vi "ME_acquire_14_DeltaForce_Daq_steppingMode.vi"() -> ()   [LabVIEW 2015]
doc: "Use this template to build a producer/consumer design pattern. Use this template when you need to execute a process, such as data analysis, when a data source, such as a triggered acquisition, produces data at an uneven rate and you need to execute the process when the data becomes available."
uses:
  Mode.ctl
  oxford_driver/Oxford Drivers/BUSGEN.LLB/OxfordAddress.ctl
  <vilib>/Analysis/baseanly.llb/Mean (DBL).vi
  <vilib>/DAQmx/read.llb/DAQmx Read (Analog 1D DBL 1Chan NSamp).vi
  <vilib>/DAQmx/create/channels.llb/DAQmx Create Channel (AI-Voltage-Basic).vi
  <vilib>/DAQmx/configure/timing.llb/DAQmx Timing (Sample Clock).vi
  <vilib>/Utility/file.llb/Write Delimited Spreadsheet (DBL).vi
  <vilib>/DAQmx/miscellaneous.llb/DAQmx Fill In Error Info.vi
  <vilib>/express/express arith-compare/Formula/XNode/ExpressFormulaBlockNode.xnode
  <vilib>/Analysis/NI_AALBase.lvlib
panel:
  out "No pol":bool=TRUE
  out "Actual2":dbl
  in  "First offset?":bool
  in  "Ready2Step":bool
  out "Last2":dbl
  out "remaining elements 2":T1(array[cluster])
  out "Actual mean":dbl format="%0.6f"
  in  "Averaged dt":dbl[][](array[numeric])
  in  "Averaged P(B)":dbl[][](array[numeric])
  out "LockInR":dbl
  out "deltaUaux":dbl
  out "Actual Voltage (V)":dbl caption="Actual AuxV" step=0.1
  in  "Stop":bool
  out "SaveSweep":bool=TRUE
  out "Measurement File_dn":path
  out "Measurement File_up":path
  out "Measurement File_average":path
  out "Actual Polarization":dbl
  in  "Reset IB?":bool
  in  "First?":bool
  in  "Save Period":dbl=1.0
  out "Averaged I(B)":dbl[][](array[numeric])
  out "P(uC/mm^2)":dbl[](array[numeric])
  in  "Sweep":bool
  out "Offset array":dbl[](array[numeric])
  in  "stop 2":bool
  in  "dB":dbl=0.005
  in  "Dwell Time (ms)":u32=1
  out "appended array":dbl[][](array[numeric])
  out "Actual B Field (T)":dbl
  out "Actual Temperature (K)":dbl
  out "Actual Current (pA)":dbl
  in  "Tab Control":T2(tab)
  in  "Max temperature (K)":dbl=20.0
  in  "Min Temperature (K)":dbl=4.5
  out "P(T)":cluster{"yi":dbl[], dbl[]}(graph)
  out "I(T)":cluster{dbl[], dbl[]}(graph)
  in  "Set temperature (K)":dbl=4.5
  in  "Temp Ramping Rate (K/min)":dbl=10.0
  in  "Heater Range":enum16{"Off", "Low", "Medium", "High"}(ring)
  in  "Heater On/Off":bool
  out "Setpoint Temperature (K)":dbl
  in  "Window (s)":dbl
  in  "Dwell Time (s)":dbl
  in  "Field Step (T)":dbl
  in  "Stepping Mode":bool
  out "I(B) 3":cluster{dbl[], dbl[]}[](graph)
  out "I(B) /Averaged/":cluster{"B array":dbl[], dbl[]}[](graph)
  out "P(B) /Averaged/":cluster{"B array":dbl[], dbl[]}[](graph)
  out "P(B)":cluster{"yi":dbl[], dbl[]}(graph)
  in  "Set Field (T)":dbl
  in  "Go to Set":bool
  in  "Sweep Rate (T/min)":dbl=2.0 format="%.6f"
  in  "Field To Zero":bool
  out "Target Field":dbl
  in  "Min Field (T)":dbl
  in  "Max Field (T)":dbl=0.15
  in  "Threshold B (T)":dbl
  out "Up/Down":bool
  in  "ReOffset":bool
  out "I(t)":dbl(graph)
  out "B(t)":dbl(graph)
  in  "Max count array":i32[](array[numeric])=[2, 1, 0, 0, 0, 9, 10, 11, 12]
  in  "secs to wait":dbl=180.0
  out "Wait (s)":dbl
  in  "Directory":string
  out "Finished":bool=TRUE
  out "Step Rate":bool
  out "New":bool=TRUE
  in  "Temperature Array":dbl[](array[numeric])=[4.5, 5.0, 6.0, 7.0, 8.0, 9.0, 10.0, 11.0, 12.0]
  in  "Sweep Rate Array":dbl[](array[numeric])=[2.0, 1.0, 0.5, 0.1, 0.05, 9.0, 10.0, 11.0, 12.0]
  in  "Record ALL":bool
  in  "Max Countl":i32
  out "i":i32
  out "j":i32
  out "Step Temp":bool
  in  "FileName":string
  in  "Measure Noise":bool
  in  "Cycles":i32
  in  "maximum value":dbl=10.0 format="%0.2f"
  in  "minimum value":dbl=-10.0 format="%0.2f"
  in  "physical channels":tag="Dev1/ai1"
  out "PSD (pA/Hz^1/2) Peaks Removed":cluster{"f0":dbl, "df":dbl, "magnitude":dbl[]}(graph)
  out "PSD (pA/Hz^1/2)":cluster{"f0":dbl, "df":dbl, "magnitude":dbl[]}(graph)
  out "Current (pA) Filtered":waveform(dbl)(graph)
  out "Current (pA)":dbl[](graph)
  in  "Samples per channel":i32=1000
  in  "Rate":dbl=1000.0 format="%0.2f"
  in  "Cut-Off Frequency":dbl=100.0 caption="Lower Cut-Off"
  in  "Filter On":bool
  in  "Lock_in_Amplifier":refnum<visa-resource-name>="GPIB0::5::INSTR"
  out "Dc offset":dbl
  in  "Calibrate":bool
  in  "IV converter":refnum<visa-resource-name>="GPIB0::20::INSTR"
  in  "Magnetic Field":refnum<visa-resource-name>="GPIB0::21::INSTR"
  out "Time Lag":dbl=0.0500025749206543
  in  "Lake Shore":refnum<visa-resource-name>="GPIB0::11::INSTR"
  in  "Temp Refresh (s)":dbl=0.1
  in  "Sampling rate (Hz)":dbl=10.0
  in  "Gain (V/A)":dbl=1000000000.0
  in  "Sample area (mm^2)":dbl=1.0
  out "B_V":cluster{dbl[], "Best Linear Fit":dbl[]}[](graph)=[{[-0.00824276058, -0.00825443003, -0.00321183179, 0.00231176104, 0.00884956705, 0.0149905744, 0.0216812607, 0.0279766336, 0.0349330416, 0.0411953716, 0.0480051807, 0.0542754057, 0.0609032504, 0.0669260394, 0.0738628706, 0.0800669926, 0.0863286519, 0.0933777995, 0.099599688, 0.107340216, 0.113761556, 0.118682905, 0.126619495, 0.134198466, 0.140806839, 0.147543465, 0.154230554, 0.161238153, 0.167889746, 0.174562307, 0.180709351, 0.186845666, 0.193431356, 0.20078938, 0.206999692, 0.213664344, 0.21973451, 0.22642957, 0.232505683, 0.23932268, 0.246070279, 0.252111494, 0.259500232, 0.265590936, 0.271561847, 0.279541147, 0.28623026, 0.292989935, 0.298956555, 0.305738485, 0.312378369, 0.319038606, 0.325861428, 0.331749698, 0.337772536, 0.344588307, 0.351860931, 0.358493458, 0.364558106, 0.37132097, 0.377974157], "Best Linear Fit"=[0.0, 0.0015, 0.0036, 0.0057, 0.0077, 0.0097, 0.0117, 0.0139, 0.0159, 0.0179, 0.0199, 0.0219, 0.0239, 0.0259, 0.0279, 0.0299, 0.032, 0.034, 0.036, 0.0381, 0.0401, 0.0423, 0.0443, 0.0463, 0.0484, 0.0505, 0.0525, 0.0545, 0.0567, 0.0587, 0.0607, 0.0627, 0.0647, 0.0668, 0.0687, 0.0707, 0.0727, 0.0747, 0.0767, 0.0788, 0.0808, 0.0828, 0.0849, 0.0869, 0.0889, 0.0911, 0.0932, 0.0952, 0.0972, 0.0993, 0.1015, 0.1035, 0.1055, 0.1075, 0.1095, 0.1115, 0.1136, 0.1156, 0.1176, 0.1197, 0.1217]}, {[-0.00824276058, -0.00825443003, -0.00321183179, 0.00231176104, 0.00884956705, 0.0149905744, 0.0216812607, 0.0279766336, 0.0349330416, 0.0411953716, 0.0480051807, 0.0542754057, 0.0609032504, 0.0669260394, 0.0738628706, 0.0800669926, 0.0863286519, 0.0933777995, 0.099599688, 0.107340216, 0.113761556, 0.118682905, 0.126619495, 0.134198466, 0.140806839, 0.147543465, 0.154230554, 0.161238153, 0.167889746, 0.174562307, 0.180709351, 0.186845666, 0.193431356, 0.20078938, 0.206999692, 0.213664344, 0.21973451, 0.22642957, 0.232505683, 0.23932268, 0.246070279, 0.252111494, 0.259500232, 0.265590936, 0.271561847, 0.279541147, 0.28623026, 0.292989935, 0.298956555, 0.305738485, 0.312378369, 0.319038606, 0.325861428, 0.331749698, 0.337772536, 0.344588307, 0.351860931, 0.358493458, 0.364558106, 0.37132097, 0.377974157], "Best Linear Fit"=[0.0023130671909174904, 0.0023094596731686335, 0.003868338853520157, 0.005575913689667713, 0.007597024472065889, 0.009495468101455781, 0.01156384061080984, 0.013510005123483607, 0.015660523385123023, 0.017596472947801402, 0.01970167132429517, 0.021640061563494486, 0.023689007091511245, 0.025550904457292693, 0.027695370706757948, 0.02961332572872314, 0.03154906794982551, 0.033728255921950154, 0.035651703316228106, 0.038044626045707346, 0.04002973228648501, 0.041551128227666274, 0.04400466196665122, 0.04634764063321815, 0.04839056663989068, 0.050473141042489685, 0.05254040147513078, 0.054706745027686375, 0.056763032153958, 0.05882580137083012, 0.060726111182603806, 0.06262310420927387, 0.0646590179467223, 0.06693369260375522, 0.0688535612150383, 0.07091388542740072, 0.07279042901630216, 0.07486015362026034, 0.07673853567696039, 0.07884595613562831, 0.08093192275399225, 0.08279951637127143, 0.08508368601736883, 0.08696657876578731, 0.0888124384600611, 0.09127917565619728, 0.09334706179235687, 0.09543676161017195, 0.09728129477588952, 0.09937787455012936, 0.10143054193208385, 0.1034895012822753, 0.10559872249341117, 0.10741903437915212, 0.10928094689289425, 0.11138798834340323, 0.11363626226897475, 0.11568665529283369, 0.11756149303587794, 0.11965217870770509, 0.12170895860641172]}]
  out "V_I":cluster{dbl[], "Best Linear Fit":dbl[]}[](graph)=[{[0.0, 0.013, 0.027, 0.041, 0.054, 0.069, 0.083, 0.098, 0.112, 0.125, 0.139, 0.153, 0.167, 0.181, 0.195, 0.208, 0.222, 0.237, 0.251, 0.265, 0.28, 0.294, 0.308, 0.322, 0.337, 0.351, 0.365, 0.379, 0.393, 0.408, 0.422, 0.435, 0.449, 0.463, 0.477, 0.491, 0.505, 0.518, 0.532, 0.547, 0.561, 0.575, 0.589, 0.603, 0.618, 0.632, 0.647, 0.66, 0.674, 0.689, 0.703, 0.718, 0.731, 0.745, 0.759, 0.773, 0.787, 0.802, 0.815, 0.829, 0.844], "Best Linear Fit"=[-0.00824276058, -0.00825443003, -0.00321183179, 0.00231176104, 0.00884956705, 0.0149905744, 0.0216812607, 0.0279766336, 0.0349330416, 0.0411953716, 0.0480051807, 0.0542754057, 0.0609032504, 0.0669260394, 0.0738628706, 0.0800669926, 0.0863286519, 0.0933777995, 0.099599688, 0.107340216, 0.113761556, 0.118682905, 0.126619495, 0.134198466, 0.140806839, 0.147543465, 0.154230554, 0.161238153, 0.167889746, 0.174562307, 0.180709351, 0.186845666, 0.193431356, 0.20078938, 0.206999692, 0.213664344, 0.21973451, 0.22642957, 0.232505683, 0.23932268, 0.246070279, 0.252111494, 0.259500232, 0.265590936, 0.271561847, 0.279541147, 0.28623026, 0.292989935, 0.298956555, 0.305738485, 0.312378369, 0.319038606, 0.325861428, 0.331749698, 0.337772536, 0.344588307, 0.351860931, 0.358493458, 0.364558106, 0.37132097, 0.377974157]}, {[0.0, 0.013, 0.027, 0.041, 0.054, 0.069, 0.083, 0.098, 0.112, 0.125, 0.139, 0.153, 0.167, 0.181, 0.195, 0.208, 0.222, 0.237, 0.251, 0.265, 0.28, 0.294, 0.308, 0.322, 0.337, 0.351, 0.365, 0.379, 0.393, 0.408, 0.422, 0.435, 0.449, 0.463, 0.477, 0.491, 0.505, 0.518, 0.532, 0.547, 0.561, 0.575, 0.589, 0.603, 0.618, 0.632, 0.647, 0.66, 0.674, 0.689, 0.703, 0.718, 0.731, 0.745, 0.759, 0.773, 0.787, 0.802, 0.815, 0.829, 0.844], "Best Linear Fit"=[-0.016453575077272017, -0.010376221021590415, -0.0038313781923948447, 0.002713464636800727, 0.008790818692482327, 0.01580315029519187, 0.02234799312438744, 0.02936032472709698, 0.03590516755629255, 0.04198252161197415, 0.04852736444116973, 0.05507220727036529, 0.061617050099560866, 0.06816189292875643, 0.074706735757952, 0.0807840898136336, 0.08732893264282918, 0.09434126424553871, 0.10088610707473429, 0.10743094990392986, 0.1144432815066394, 0.12098812433583496, 0.12753296716503054, 0.1340778099942261, 0.14109014159693567, 0.1476349844261312, 0.15417982725532678, 0.16072467008452238, 0.16726951291371794, 0.17428184451642745, 0.18082668734562304, 0.18690404140130465, 0.19344888423050022, 0.19999372705969579, 0.20653856988889135, 0.21308341271808692, 0.2196282555472825, 0.2257056096029641, 0.2322504524321597, 0.23926278403486922, 0.2458076268640648, 0.2523524696932603, 0.2588973125224559, 0.2654421553516515, 0.27245448695436103, 0.2789993297835566, 0.28601166138626616, 0.29208901544194776, 0.29863385827114336, 0.30564618987385284, 0.31219103270304843, 0.31920336430575796, 0.32528071836143957, 0.3318255611906351, 0.3383704040198307, 0.3449152468490263, 0.35146008967822184, 0.35847242128093143, 0.364549775336613, 0.3710946181658085, 0.3781069497685181]}]
  out "B0 (T)":dbl=0.004861251132056582
  out "B/V (T/V)":dbl=0.30914205458325855
  out "I0 (A)":dbl=-0.016453575077272017
  out "V/I (Ohm)":dbl=0.46748877351396934
  in  "Offset?":bool
  in  "Magnet":bool
  in  "Ramp":bool=TRUE
  in  "DaQ":bool
  in  "Moving average":i8=10
  in  "Sample Rate":dbl=1000.0
  in  "Number of Samples":i32=100
  in  "Physical Channel":tag="kartya/ai0"
  in  "Min Voltage":dbl=-5.0
  in  "Max Voltage":dbl=5.0
  in  "Terminal Configuration":i32(ring)=-1 items=["default"=-1, "RSE"=10083, "NRSE"=10078, "Differential"=10106, "Pseudodifferential"=12529]
  in  "Count":i32=100
  in  "Temp/Magnetic Field":bool
  out "index":i8
  out "Read?":bool
  out "Magnetic Field (T)":dbl[](array[numeric])
  out "Reset":bool
  out "Measured Current (pA)":dbl[](array[numeric])
  out "Elapsed Time (s)":dbl[](array[numeric])
  out "Start time":timestamp
  in  "Enum":T3=enum."Process"
  out "B array":dbl[](array[numeric])
  in  "dB (T)":dbl=0.0025
  in  "Counter":i8
  out "L magnet (H)":dbl
  out "R magnet (mOhm)":dbl
  out "Actual Current (R0)":dbl
  out "Actual Field (T)":dbl
  out "Temperature array":dbl[](array[numeric])
  in  "New Measurement File":bool
  out "Measurement File":path
  out "refnum out":refnum<file>
  in  "Measuring":bool
  in  "Measure /Pause":bool
  in  "stop":bool
  # "DeltaForce"
  # "Discrete"
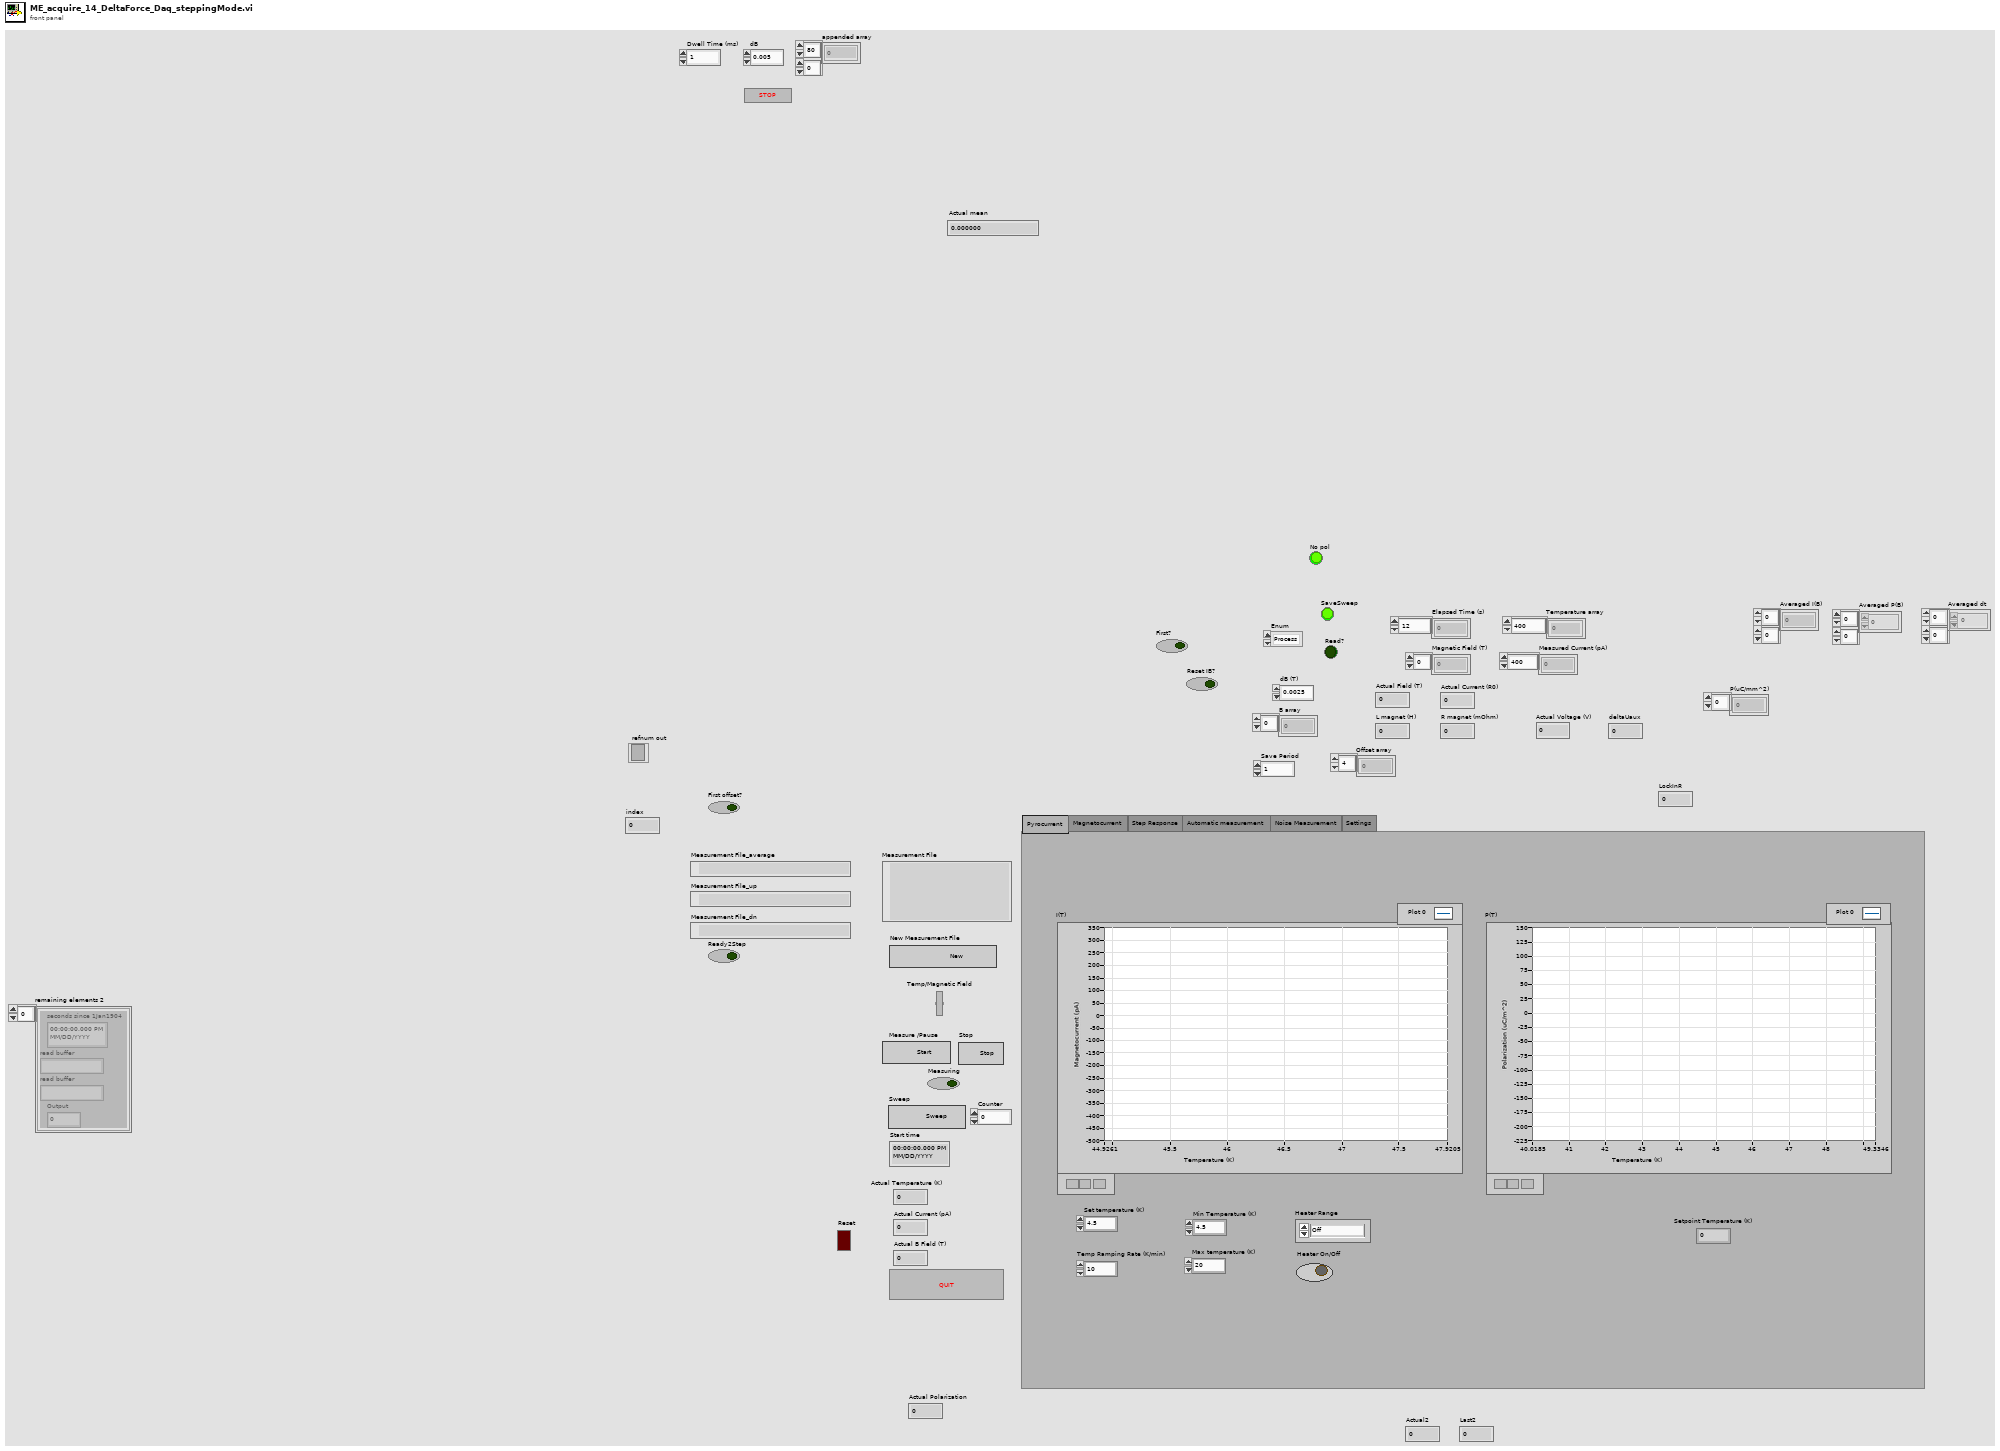
[diagram p1: front panel]
types:
  T1 = cluster{"seconds since 1Jan1904":timestamp, "read buffer":string, "read buffer":string, "Output":dbl}[]
  T2 = enum32{"Pyrocurrent", "Magnetocurrent", "Step Response", "Automatic measurement", "Noise Measurement", "Settings"}
  T3 = typedef "Mode.ctl" = enum16{"Offset", "Process", "Sweep", "StepOxford", "StepDelta", "Plot", "Save", "New", "Return", ""}
  T4 = cluster{"seconds since 1Jan1904":timestamp, "read buffer":string, "read buffer":string, "Output":dbl}
  T5 = enum16{"open", "replace", "create", "open or create", "replace or create", "replace or create with confirmation"}
  T6 = typedef "OxfordAddress.ctl" = cluster{"Com Port":i32, "ISOBUS Address":i32, "GPIB Address":i16, "Communication":enum16{"RS232", "ISOBUS", "GPIB", "Gateway"}}
  T7 = cluster{"B array":dbl[], "Averaged P(B) Out":dbl[]}
  T8 = cluster{"B array":dbl[], "BaselineSubtracted I(B)":dbl[]}
  T9 = cluster{"B array":dbl[], "Averaged P(B) Out":dbl[]}[]
  T10 = cluster{"B array":dbl[], "BaselineSubtracted I(B)":dbl[]}[]
  T11 = cluster{"I array out (A)":dbl[], "V array out (V)":dbl[]}
  T12 = cluster{"I array out (A)":dbl[], "Best Linear Fit":dbl[]}
  T13 = cluster{"V array out (V)":dbl[], "B array Out":dbl[]}
  T14 = cluster{"V array out (V)":dbl[], "Best Linear Fit 2":dbl[]}
  T15 = cluster{"I array out (A)":dbl[], "Best Linear Fit":dbl[]}[]
  T16 = cluster{"V array out (V)":dbl[], "Best Linear Fit 2":dbl[]}[]
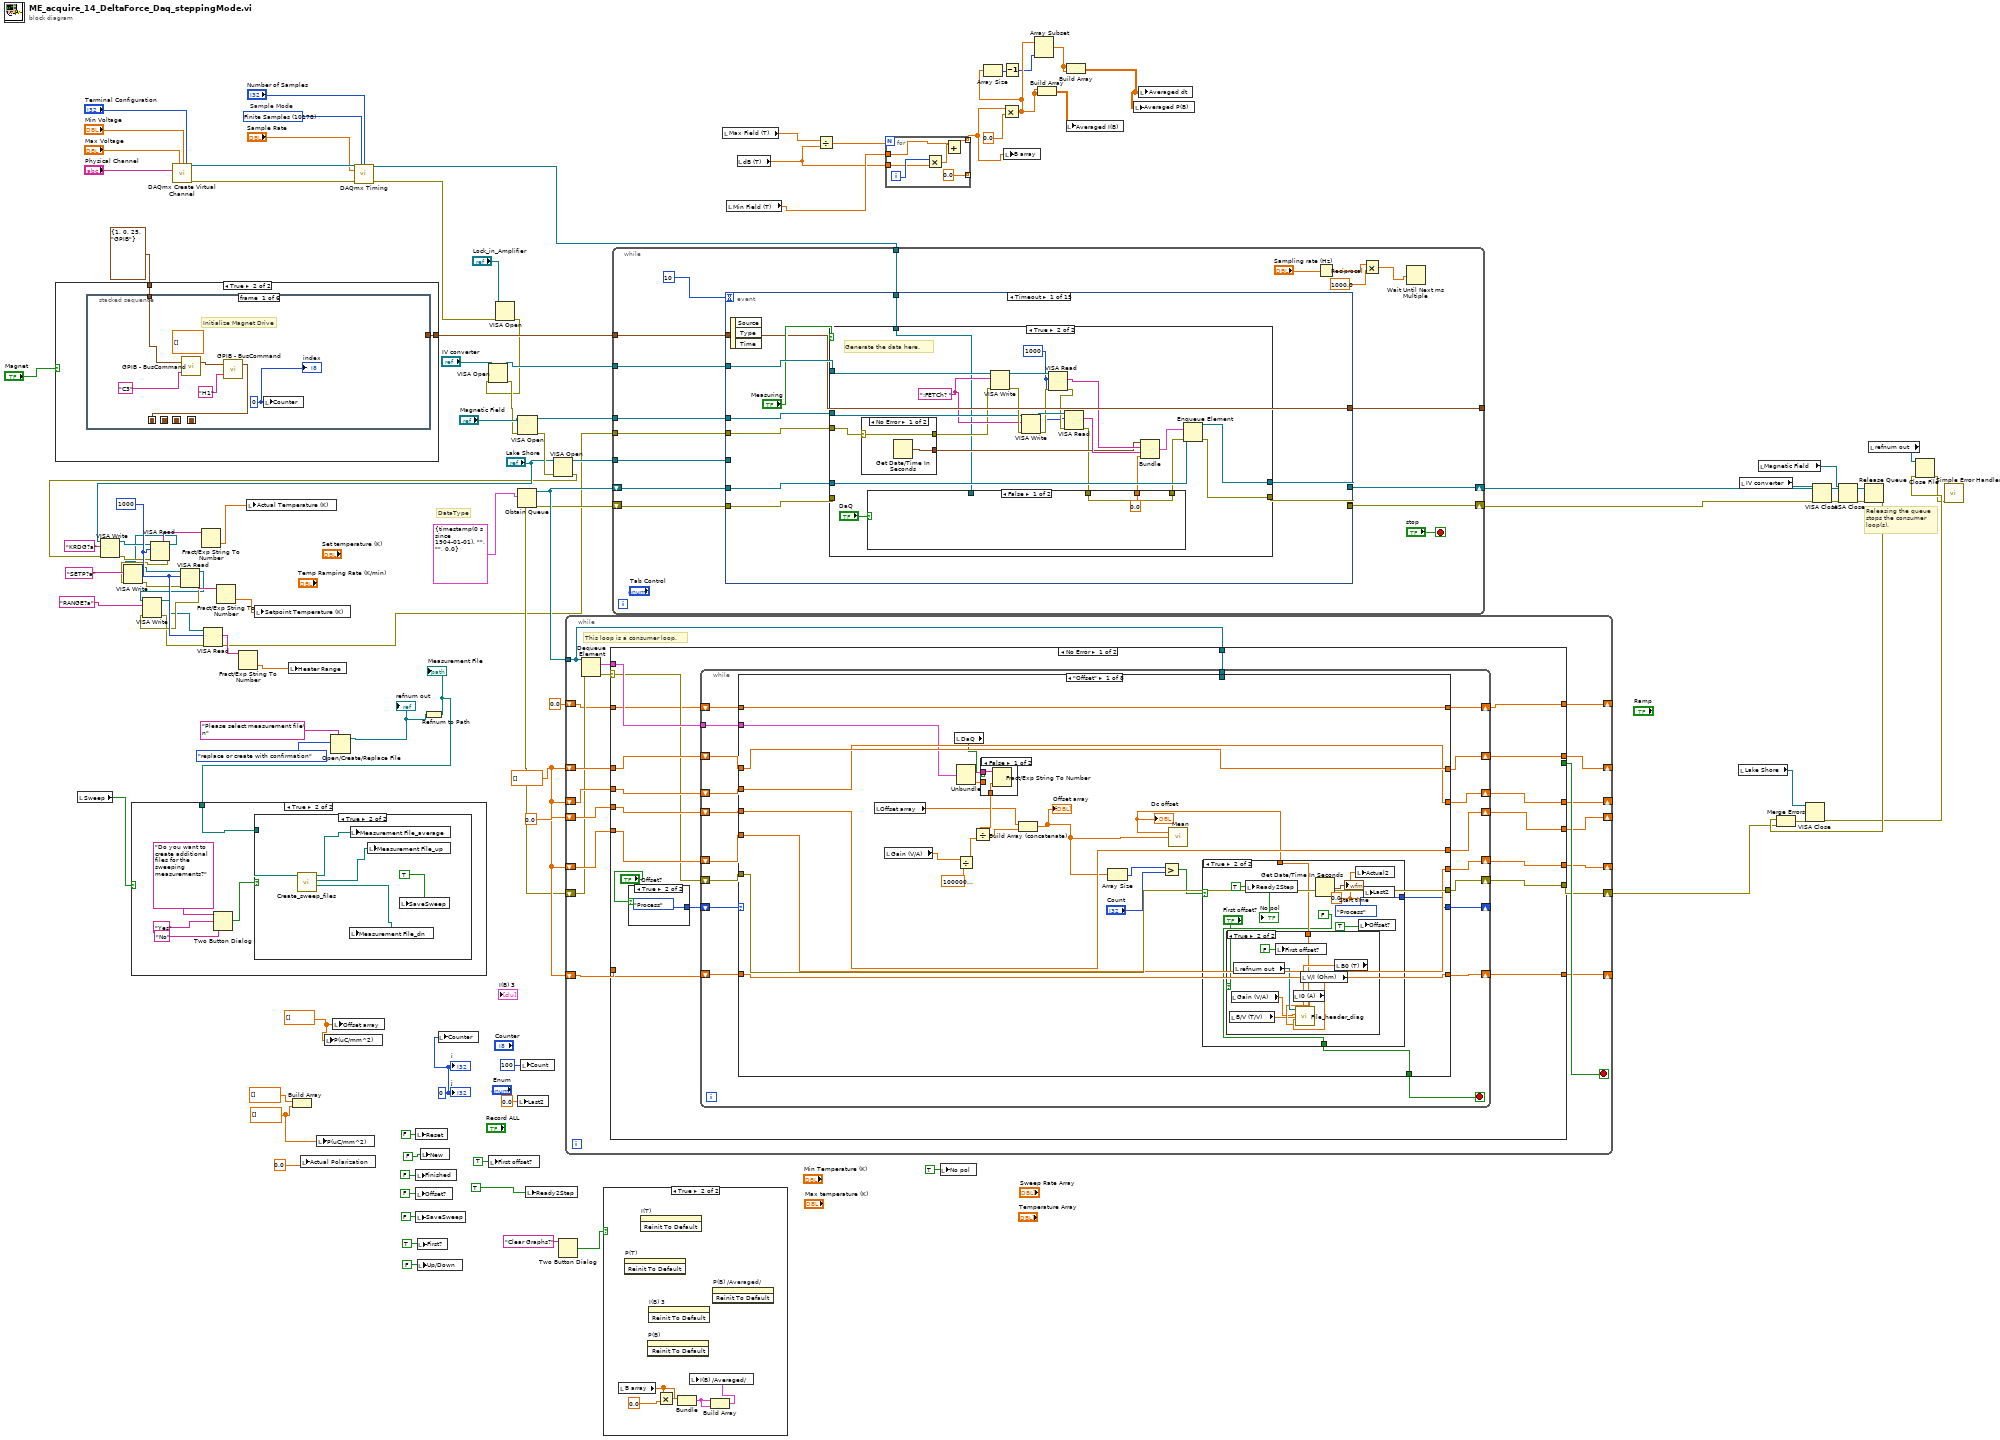
[diagram p0: block diagram]
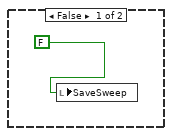
[diagram p4: hidden frame]
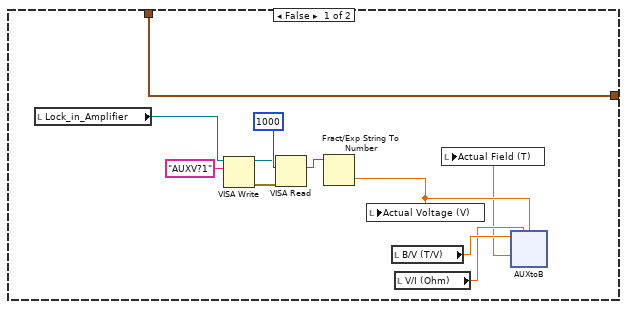
[diagram p5: hidden frame]
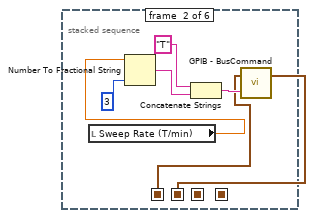
[diagram p6: hidden frame]
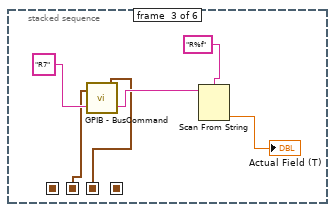
[diagram p7: hidden frame]
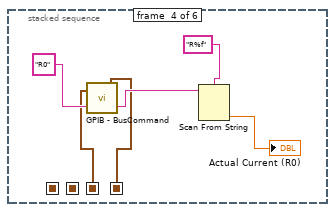
[diagram p8: hidden frame]
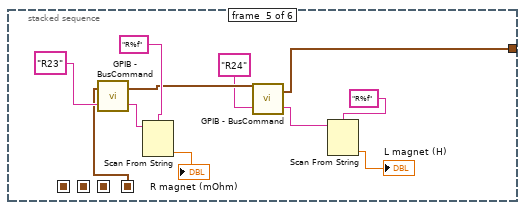
[diagram p9: hidden frame]
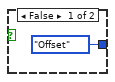
[diagram p11: hidden frame]
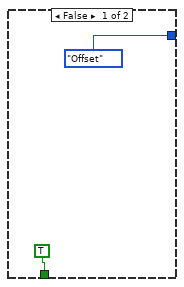
[diagram p13: hidden frame]
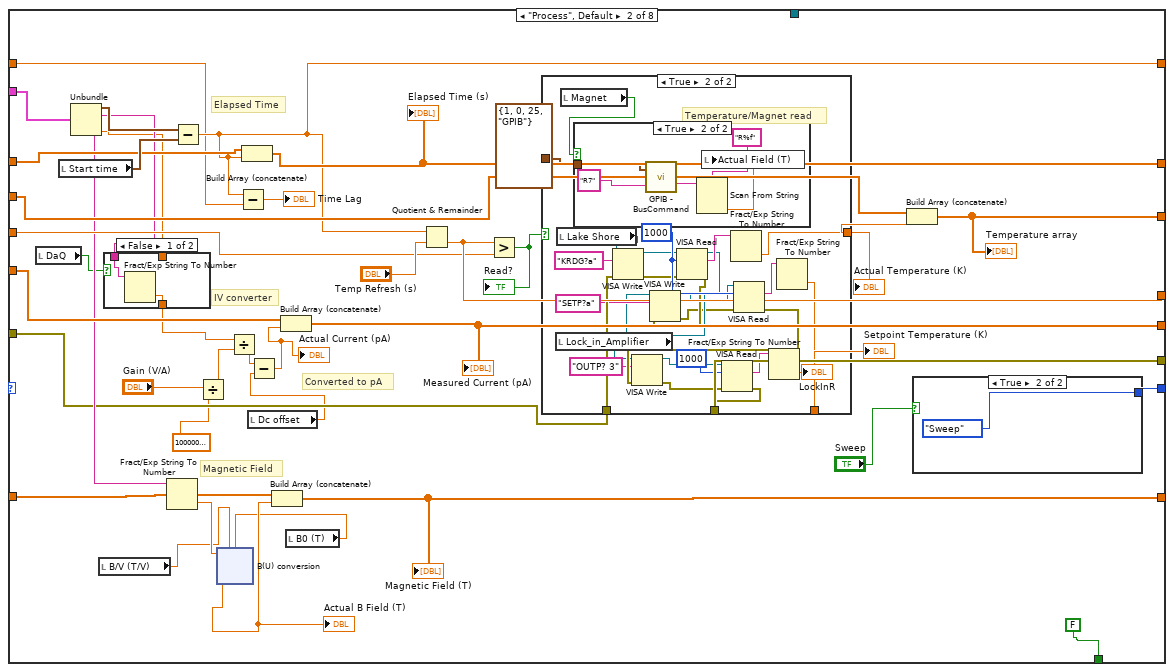
[diagram p15: hidden frame]
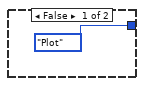
[diagram p17: hidden frame]
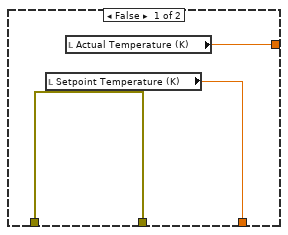
[diagram p18: hidden frame]
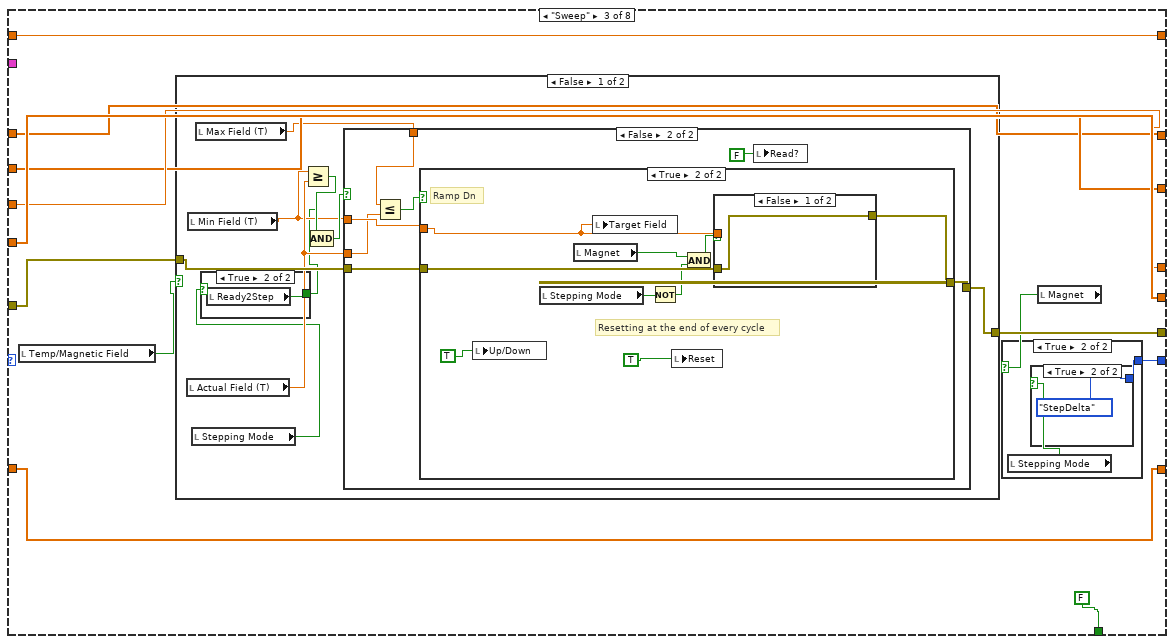
[diagram p20: hidden frame]
diagram:
  w17 = 10178 items=["Finite Samples"=10178, "Continuous Samples"=10123, "Hardware Timed Single Point"=12522]  # Sample Mode
  w44 = u32 1000 ("byte count")
  w55 = 0 ("j")
  w52 = dbl[] []
  w70 = dbl[] []
  w76 = dbl[] []
  # "DataType"
  # "Releasing the queue stops the consumer loop(s)."
  n1 = case shown="True" "Magnet" {
    tunnel: T6 {"Com Port"=1, "ISOBUS Address"=0, "GPIB Address"=25, "Communication"=enum."GPIB"} ("Address") -> [w112 w126]
    tunnel: [w112 w125] -> w82
    frame False {
      n2 = local read "Lock_in_Amplifier"() -> (w106:refnum<visa-resource-name>)
      n3 = VISA Write(VISA resource name=w106, write buffer="AUXV?1") -> (VISA resource name out=w107:refnum<visa-resource-name>, error out=w111:errorcluster)  [unwired: 1 in, 1 out]
      n4 = VISA Read(VISA resource name=w107, byte count=u32 1000, error in (no error)=w111) -> (read buffer=w110:string)  [unwired: 3 out]
      n5 = Fract/Exp String To Number(string=w110) -> (number=w103:dbl)  [unwired: 3 in, 1 out]
      n6 = local write "Actual Voltage (V)"(w103) -> ()
      n7 = local read "B/V (T/V)"() -> (w105:dbl)
      n8 = local read "V/I (Ohm)"() -> (w104:dbl)
      n9 = xnode "AUXtoB"("BpV"=w105, "Rm"=w104, "Aux"=w103) -> ("Result"=w102:dbl)  [unwired: 1 in, 1 out]
      n10 = local write "Actual Field (T)"(w102) -> ()
    }
    frame True {
      n11 = stacked-sequence {
        seq-local: [w129 _ _ _ _ _] -> [_ w134 _ _ _ _]
        seq-local: [_ w133 _ _ _ _] -> [_ _ w141 _ _ _]
        seq-local: [_ _ w140 _ _ _] -> [_ _ _ w147 _ _]
        seq-local: [_ _ _ w146 _ _] -> [_ _ _ _ w158 _]
        tunnel: w126 -> [w131 _ _ _ _ _]
        tunnel: [_ _ _ _ w156 _] -> w125
        frame #0 {
          (unwired) dbl[][] []
          w127 = i8 0 ("Counter")
          # "Initialize Magnet Drive"
          n12 = call "GPIB - BusCommand.vi"("Command"="C3", "Address"=w131) -> ("Address(thru)"=w130:T6)  [unwired: 1 out]
          n13 = call "GPIB - BusCommand.vi"("Command"="H1", "Address"=w130) -> ("Address(thru)"=w129:T6)  [unwired: 1 out]
          n14 = local write "Counter"(w127) -> ()
          "index" <- w127
        }
        frame #1 {
          n15 = local read "Sweep Rate (T/min)"() -> (w135:dbl)
          n16 = Number To Fractional String(number=w135, precision (6)=i16 3) -> (F-format string=w137:string)  [unwired: 2 in]
          n17 = Concatenate Strings("T" ("format string"), w137) -> (w136:string)
          n18 = call "GPIB - BusCommand.vi"("Command"=w136, "Address"=w134) -> ("Address(thru)"=w133:T6)  [unwired: 1 out]
        }
        frame #2 {
          n19 = call "GPIB - BusCommand.vi"("Command"="R7" ("format string"), "Address"=w141) -> ("Reply"=w145:string, "Address(thru)"=w140:T6)
          n20 = Scan From String(format string="R%f" ("remaining string"), input string=w145) -> (output 1=→"Actual Field (T)":dbl)  [unwired: 3 in, 3 out]
        }
        frame #3 {
          n21 = call "GPIB - BusCommand.vi"("Command"="R0" ("format string"), "Address"=w147) -> ("Reply"=w151:string, "Address(thru)"=w146:T6)
          n22 = Scan From String(format string="R%f" ("remaining string"), input string=w151) -> (output 1=→"Actual Current (R0)":dbl)  [unwired: 3 in, 3 out]
        }
        frame #4 {
          n23 = call "GPIB - BusCommand.vi"("Command"="R23" ("format string"), "Address"=w158) -> ("Reply"=w162:string, "Address(thru)"=w157:T6)
          n24 = Scan From String(format string="R%f" ("remaining string"), input string=w162) -> (output 1=→"R magnet (mOhm)":dbl)  [unwired: 3 in, 3 out]
          n25 = call "GPIB - BusCommand.vi"("Command"="R24" ("format string"), "Address"=w157) -> ("Reply"=w154:string, "Address(thru)"=w156:T6)
          n26 = Scan From String(format string="R%f" ("remaining string"), input string=w154) -> (output 1=→"L magnet (H)":dbl)  [unwired: 3 in, 3 out]
        }
        frame #5 {
        }
      }
    }
  }
  n27 = local read "Sweep"() -> (w60:bool)
  n28 = call-poly <vilib>:"DAQmx Create Virtual Channel.vi"("maximum value"="Max Voltage", "minimum value"="Min Voltage", "input terminal configuration"="Terminal Configuration", "physical channels"="Physical Channel") -> ("task out"=w15:refnum<k21>, "error out"=w16:errorcluster)  [unwired: 10 in]
  n29 = Build Array(dbl[] [], w52) -> ()  [unwired: 1 out]
  n30 = local write "Actual Polarization"(0.0 ("Actual Polarization")) -> ()
  n31 = local write "P(uC/mm^2)"(w52) -> ()
  n32 = local write "P(uC/mm^2)"(w70) -> ()
  n33 = Open/Create/Replace File(prompt="Please select measurement file\n", operation (0:open)=T5."replace or create with confirmation") -> (refnum out=w79:refnum<file>)  [unwired: 4 in, 2 out]
  "refnum out" <- w79
  n34 = local write "Offset array"(w70) -> ()
  n35 = call-poly <vilib>:"DAQmx Timing.vi"("task/channels in"=w15, "sample mode"=w17, "samples per channel"="Number of Samples", "rate"="Sample Rate", "error in"=w16) -> ("task out"=w7:refnum<k21>, "error out"=w8:errorcluster)  [unwired: 9 in]
  n36 = local write "Finished"(FALSE ("Finished")) -> ()
  n37 = local write "Offset?"(FALSE ("Offset?")) -> ()
  n38 = local write "Reset"(FALSE ("Reset")) -> ()
  n39 = local write "SaveSweep"(FALSE ("SaveSweep")) -> ()
  n40 = local write "First?"(TRUE ("First?")) -> ()
  n41 = local write "Up/Down"(FALSE ("Up/Down")) -> ()
  n42 = local write "New"(FALSE ("New")) -> ()
  n43 = Refnum to Path(1:w79) -> (0:w59:path)
  "Measurement File" <- w59
  n44 = case shown="True" w60 {
    tunnel: w59 -> [_ w163]
    frame False {
    }
    frame True {
      n45 = Two Button Dialog(message="Do you want to create additional files for the sweeping measurements?" ("string"), 1:"No" ("F button name (\"Cancel\")"), 2:"Yes" ("T button name (\"OK\")")) -> (T button?=w165:bool)
      n46 = case shown="True" w165 {
        tunnel: w163 -> [_ w173]
        frame False {
          n47 = local write "SaveSweep"(FALSE ("SaveSweep")) -> ()
        }
        frame True {
          n48 = call "Create_sweep_files.vi"("Measurement File"=w173) -> ("Path 3"=w170:path, "Path 2"=w171:path, "Path"=w172:path)  [unwired: 8 in]
          n49 = local write "Measurement File_dn"(w170) -> ()
          n50 = local write "Measurement File_average"(w172) -> ()
          n51 = local write "Measurement File_up"(w171) -> ()
          n52 = local write "SaveSweep"(TRUE) -> ()
        }
      }
    }
  }
  n53 = local write "Counter"(w55) -> ()
  n54 = local write "First offset?"(TRUE ("First offset?")) -> ()
  n55 = VISA Open(error in (no error)=w8, VISA resource name="Lock_in_Amplifier") -> (error out=w27:errorcluster)  [unwired: 3 in, 1 out]
  n56 = VISA Open(error in (no error)=w27, VISA resource name="IV converter") -> (VISA resource name=w96:refnum<visa-resource-name>, error out=w98:errorcluster)  [unwired: 3 in]
  n57 = Obtain Queue(element data type=T4 {"seconds since 1Jan1904"=timestamp(0 s since 1904-01-01), "read buffer"="", "read buffer"="", "Output"=0.0} ("output cluster")) -> (queue out=w101:refnum<queue>, error out=w74:errorcluster)  [unwired: 4 in, 1 out]
  n58 = VISA Open(error in (no error)=w98, VISA resource name="Magnetic Field") -> (VISA resource name=w95:refnum<visa-resource-name>, error out=w77:errorcluster)  [unwired: 3 in]
  n59 = local write "Last2"(0.0 ("Last2")) -> ()
  n60 = local write "Count"(100 ("Count")) -> ()
  n61 = local write "Ready2Step"(TRUE ("Ready2Step")) -> ()
  n62 = VISA Open(error in (no error)=w77, VISA resource name="Lake Shore") -> (VISA resource name=w72:refnum<visa-resource-name>, error out=w41:errorcluster)  [unwired: 3 in]
  n63 = VISA Write(VISA resource name="Lake Shore", write buffer="KRDG?a", error in (no error)=w41) -> (VISA resource name out=w38:refnum<visa-resource-name>, error out=w37:errorcluster)  [unwired: 1 out]
  n64 = VISA Read(VISA resource name=w38, byte count=w44, error in (no error)=w37) -> (VISA resource name out=w35:refnum<visa-resource-name>, read buffer=w49:string, error out=w36:errorcluster)  [unwired: 1 out]
  n65 = VISA Write(VISA resource name=w35, write buffer="SETP?a", error in (no error)=w36) -> (VISA resource name out=w34:refnum<visa-resource-name>, error out=w33:errorcluster)  [unwired: 1 out]
  n66 = VISA Read(VISA resource name=w34, byte count=w44, error in (no error)=w33) -> (VISA resource name out=w31:refnum<visa-resource-name>, read buffer=w48:string, error out=w32:errorcluster)  [unwired: 1 out]
  n67 = VISA Write(VISA resource name=w31, write buffer="RANGE?a", error in (no error)=w32) -> (VISA resource name out=w29:refnum<visa-resource-name>, error out=w30:errorcluster)  [unwired: 1 out]
  n68 = Fract/Exp String To Number(string=w49) -> (number=w47:dbl)  [unwired: 3 in, 1 out]
  n69 = VISA Read(VISA resource name=w29, byte count=w44, error in (no error)=w30) -> (read buffer=w43:string, error out=w40:errorcluster)  [unwired: 2 out]
  n70 = Fract/Exp String To Number(string=w48) -> (number=w46:dbl)  [unwired: 3 in, 1 out]
  n71 = Fract/Exp String To Number(string=w43) -> (number=w39:dbl)  [unwired: 3 in, 1 out]
  n72 = local write "Actual Temperature (K)"(w47) -> ()
  n73 = local write "Setpoint Temperature (K)"(w46) -> ()
  n74 = local write "Heater Range"(w39) -> ()
  n75 = Two Button Dialog(message="Clear Graphs?") -> (T button?=w54:bool)  [unwired: 2 in]
  n76 = while {
    tunnel: w101 -> [w174]
    shift-right: [w187] -> _
    shift-left: w76 -> [w186]
    shift-right: [w185] -> _
    shift-left: w76 -> [w184]
    shift-right: [w183] -> _
    shift-left: w76 -> [w182]
    shift-right: [w181] -> _
    shift-left: 0.0 -> [w180]
    shift-right: [w179] -> _
    shift-left: w76 -> [w178]
    shift-right: [w188] -> w87
    shift-left: w74 -> [w177]
    shift-right: [w176] -> _
    shift-left: 0.0 -> [w175]
    stop <- w189 stop-if-true
    # "This loop is a consumer loop."
    n77 = Dequeue Element(queue=w174, error in (no error)=w177) -> (element=w190:T4, error out=w191:errorcluster)  [unwired: 1 in, 2 out]
    n78 = case shown="No Error" w191 {
      selector: w191 -> [w197 w938]
      tunnel: w190 -> [w208 _]
      tunnel: [_ TRUE] -> w189
      tunnel: [w196 w938] -> w188
      tunnel: [w207 w937] -> w187
      tunnel: w186 -> [w206 w937]
      tunnel: [w205 w934] -> w185
      tunnel: w184 -> [w204 w934]
      tunnel: [w203 w933] -> w183
      tunnel: w182 -> [w202 w933]
      tunnel: [w201 w935] -> w181
      tunnel: w180 -> [w200 w935]
      tunnel: [w199 w936] -> w179
      tunnel: w178 -> [w198 w936]
      tunnel: [w195 w932] -> w176
      tunnel: w175 -> [w194 w932]
      tunnel: w174 -> [w192 _]
      frame No Error {
        n79 = case shown="True" "Offset?" {
          tunnel: [Mode."Offset" ("Enum") Mode."Process" ("Enum")] -> w209
          frame False {
          }
          frame True {
          }
        }
        n80 = while {
          shift-right: [w218] -> _
          shift-left: w209 -> [w230]
          tunnel: w208 -> [w229]
          shift-right: [w228] -> w207
          shift-left: w206 -> [w227]
          shift-right: [w220] -> w199
          shift-left: w198 -> [w219]
          shift-right: [w222] -> w201
          shift-left: w200 -> [w221]
          shift-right: [w226] -> w205
          shift-left: w204 -> [w225]
          shift-right: [w216] -> w196
          shift-left: w197 -> [w217]
          shift-right: [w224] -> w203
          shift-left: w202 -> [w223]
          shift-right: [w214] -> w195
          shift-left: w194 -> [w213]
          tunnel: w192 -> [w212]
          stop <- w215 stop-if-true
          n81 = case shown="\"Offset\"" w230 {
            selector: w230 -> [_ _ _ _ _ _ _ w925]
            tunnel: w229 -> [w248 w314 _ _ _ _ _ _]
            tunnel: [w254 w311 w372 w500 w603 w683 w766 w930] -> w228
            tunnel: w227 -> [w254 w304 w372 w500 w603 w679 w766 w930]
            tunnel: [w249 w310 w375 w497 w605 w685 w764 w927] -> w226
            tunnel: w225 -> [w249 w309 w375 w497 w605 w680 w764 w927]
            tunnel: [w250 w308 w377 w496 w600 w686 w762 w924] -> w224
            tunnel: w223 -> [w250 w307 w377 w496 w600 w681 w762 w924]
            tunnel: [w252 w303 w374 w498 w601 w689 0.0 w928] -> w222
            tunnel: w221 -> [w252 w302 w374 w498 w601 w689 _ w928]
            tunnel: [w253 w299 w373 w499 w602 w684 w765 w929] -> w220
            tunnel: w219 -> [w253 w300 w373 w499 w602 w682 w765 w929]
            tunnel: [w237 w297 w370 w490 Mode."Save" ("Enum") w690 Mode."Return" ("Enum") w925] -> w218
            tunnel: w217 -> [w251 w295 w379 w494 w608 w688 w758 w926]
            tunnel: [w251 w294 w378 w493 w608 w688 w757 w926] -> w216
            tunnel: [w233 FALSE FALSE FALSE FALSE w677 TRUE TRUE] -> w215
            tunnel: [w236 w291 w371 w491 w604 w687 0.0 w931] -> w214
            tunnel: w213 -> [w236 w290 w371 w491 w604 w687 _ w931]
            tunnel: w212 -> [_ _ _ _ _ _ w756 _]
            frame "Offset" {
              n82 = local read "Offset array"() -> (w242:dbl[])
              n83 = local read "Gain (V/A)"() -> (w246:dbl)
              n84 = local read "DaQ"() -> (w232:bool)
              n85 = Unbundle(w248) -> ("read buffer"=w235:string, "Output"=w231:dbl)  [unwired: 2 out]
              n86 = Divide(x=w246, y=1000000000000.0) -> (x/y=w244:dbl)
              n87 = case shown="False" w232 {
                tunnel: [w256 w257] -> w247
                tunnel: w235 -> [w255 _]
                tunnel: w231 -> [_ w257]
                frame False {
                  n88 = Fract/Exp String To Number(string=w255) -> (number=w256:dbl)  [unwired: 3 in, 1 out]
                }
                frame True {
                }
              }
              n89 = Divide(x=w247, y=w244) -> (x/y=w243:dbl)
              n90 = Build Array (concatenate)(w242, w243) -> (w238:dbl[])
              "Offset array" <- w238
              n91 = Array Size(array=w238) -> (size(s)=w241:i32)
              n92 = Greater?(x=w241, y="Count") -> (0:w239:bool)
              n93 = call-poly <vilib>:"Mean.vi"("X"=w238) -> ("mean"=w234:dbl)  [unwired: 1 out]
              "Dc offset" <- w234
              n94 = case shown="True" w239 {
                tunnel: [Mode."Offset" ("Enum") Mode."Process" ("Enum")] -> w237
                tunnel: w234 -> [_ w266]
                tunnel: [TRUE FALSE] -> w233
                frame False {
                }
                frame True {
                  w260 = 0.0 ("Last2")
                  w261 = TRUE ("Ready2Step")
                  n95 = case shown="True" "First offset?" {
                    tunnel: w266 -> [_ w269]
                    frame False {
                    }
                    frame True {
                      n96 = local read "B/V (T/V)"() -> (w270:dbl)
                      n97 = local read "Gain (V/A)"() -> (w271:dbl)
                      n98 = local read "refnum out"() -> (w275:refnum<file>)
                      n99 = local write "First offset?"(FALSE ("First offset?")) -> ()
                      n100 = local read "I0 (A)"() -> (w273:dbl)
                      n101 = local read "V/I (Ohm)"() -> (w274:dbl)
                      n102 = local read "B0 (T)"() -> (w272:dbl)
                      n103 = call "File_header_diag.vi"("OFFSET"=w269, "B0"=w272, "B/V"=w270, "I0"=w273, "V/I"=w274, "Gain"=w271, "Byte Stream File in"=w275) -> ()  [unwired: 5 in]
                    }
                  }
                  n104 = local write "Ready2Step"(w261) -> ()
                  n105 = Get Date/Time In Seconds() -> (seconds since 1Jan1904=→"Start time":timestamp)
                  n106 = local write "Actual2"(w260) -> ()
                  n107 = local write "Offset?"(TRUE ("Offset?")) -> ()
                  n108 = local write "Last2"(w260) -> ()
                  "No pol" <- w261
                }
              }
            }
            frame "Process", Default {
              # "Converted to pA"
              # "Magnetic Field"
              # "IV converter"
              # "Elapsed Time"
              n109 = local read "DaQ"() -> (w278:bool)
              n110 = local read "Start time"() -> (w312:timestamp)
              n111 = Unbundle(w314) -> ("seconds since 1Jan1904"=w313:timestamp, "read buffer"=w279:string, "read buffer"=w296:string, "Output"=w276:dbl)
              n112 = local read "B/V (T/V)"() -> (w286:dbl)
              n113 = case shown="False" w278 {
                tunnel: w279 -> [w318 _]
                tunnel: [w317 w319] -> w277
                tunnel: w276 -> [_ w319]
                frame False {
                  n114 = Fract/Exp String To Number(string=w318) -> (number=w317:dbl)  [unwired: 3 in, 1 out]
                }
                frame True {
                }
              }
              n115 = Fract/Exp String To Number(string=w296) -> (number=w306:dbl)  [unwired: 3 in, 1 out]
              n116 = Subtract(x=w313, y=w312) -> (x-y=w291:dbl)
              n117 = Divide(x="Gain (V/A)", y=1000000000000.0) -> (x/y=w289:dbl)
              n118 = Divide(x=w277, y=w289) -> (x/y=w284:dbl)
              n119 = Subtract(x=w291, y=w290) -> (x-y=→"Time Lag":dbl)
              n120 = Build Array (concatenate)(w304, w291) -> (w311:dbl[])
              "Elapsed Time (s)" <- w311
              n121 = local read "Dc offset"() -> (w282:dbl)
              n122 = Subtract(x=w284, y=w282) -> (x-y=w283:dbl)
              "Actual Current (pA)" <- w283
              n123 = Build Array (concatenate)(w309, w283) -> (w310:dbl[])
              "Measured Current (pA)" <- w310
              n124 = local read "B0 (T)"() -> (w285:dbl)
              n125 = xnode "B(U) conversion"("V"=w306, "BpV"=w286, "B0"=w285) -> ("Result"=w305:dbl)  [unwired: 1 in, 1 out]
              "Actual B Field (T)" <- w305
              n126 = Build Array (concatenate)(w307, w305) -> (w308:dbl[])
              "Magnetic Field (T)" <- w308
              n127 = Quotient & Remainder(x=w291, y="Temp Refresh (s)") -> (floor(x/y)=w303:dbl)  [unwired: 1 out]
              n128 = Greater?(x=w303, y=w302) -> (0:w301:bool)
              "Read?" <- w301
              n129 = case shown="True" w301 {
                tunnel: [w323 w348] -> w298
                tunnel: w295 -> [w324 w347]
                tunnel: [w324 w327] -> w294
                tunnel: T6 {"Com Port"=1, "ISOBUS Address"=0, "GPIB Address"=25, "Communication"=enum."GPIB"} ("Address") -> [_ w346]
                tunnel: [w322 w342] -> w280
                frame False {
                  n130 = local read "Setpoint Temperature (K)"() -> (w322:dbl)
                  n131 = local read "Actual Temperature (K)"() -> (w323:dbl)
                }
                frame True {
                  w343 = u32 1000 ("byte count")
                  # "Temperature/Magnet read"
                  n132 = local read "Lock_in_Amplifier"() -> (w331:refnum<visa-resource-name>)
                  n133 = local read "Lake Shore"() -> (w345:refnum<visa-resource-name>)
                  n134 = local read "Magnet"() -> (w334:bool)
                  n135 = case shown="True" w334 {
                    tunnel: w346 -> [_ w352]
                    frame False {
                    }
                    frame True {
                      n136 = call "GPIB - BusCommand.vi"("Command"="R7" ("format string"), "Address"=w352) -> ("Reply"=w353:string)  [unwired: 1 out]
                      n137 = Scan From String(format string="R%f" ("remaining string"), input string=w353) -> (output 1=w351:dbl)  [unwired: 3 in, 3 out]
                      n138 = local write "Actual Field (T)"(w351) -> ()
                    }
                  }
                  n139 = VISA Write(VISA resource name=w345, write buffer="KRDG?a", error in (no error)=w347) -> (VISA resource name out=w341:refnum<visa-resource-name>, error out=w339:errorcluster)  [unwired: 1 out]
                  n140 = VISA Read(VISA resource name=w341, byte count=w343, error in (no error)=w339) -> (VISA resource name out=w340:refnum<visa-resource-name>, read buffer=w349:string, error out=w338:errorcluster)  [unwired: 1 out]
                  n141 = VISA Write(VISA resource name=w340, write buffer="SETP?a", error in (no error)=w338) -> (VISA resource name out=w336:refnum<visa-resource-name>, error out=w337:errorcluster)  [unwired: 1 out]
                  n142 = Fract/Exp String To Number(string=w349) -> (number=w348:dbl)  [unwired: 3 in, 1 out]
                  n143 = VISA Read(VISA resource name=w336, byte count=w343, error in (no error)=w337) -> (read buffer=w335:string, error out=w333:errorcluster)  [unwired: 2 out]
                  n144 = VISA Write(VISA resource name=w331, write buffer="OUTP? 3", error in (no error)=w333) -> (VISA resource name out=w330:refnum<visa-resource-name>, error out=w332:errorcluster)  [unwired: 1 out]
                  n145 = VISA Read(VISA resource name=w330, byte count=u32 1000, error in (no error)=w332) -> (read buffer=w326:string, error out=w327:errorcluster)  [unwired: 2 out]
                  n146 = Fract/Exp String To Number(string=w326) -> (number=→"LockInR":dbl)  [unwired: 3 in, 1 out]
                  n147 = Fract/Exp String To Number(string=w335) -> (number=w342:dbl)  [unwired: 3 in, 1 out]
                }
              }
              "Actual Temperature (K)" <- w298
              "Setpoint Temperature (K)" <- w280
              n148 = Build Array (concatenate)(w300, w298) -> (w299:dbl[])
              "Temperature array" <- w299
              n149 = case shown="True" "Sweep" {
                tunnel: [Mode."Plot" ("Enum") Mode."Sweep" ("Enum")] -> w297
                frame False {
                }
                frame True {
                }
              }
            }
            frame "Sweep" {
              n150 = local read "Temp/Magnetic Field"() -> (w369:bool)
              n151 = case shown="False" w369 {
                tunnel: w379 -> [w392 w457]
                tunnel: [w391 w456] -> w378
                frame False {
                  n152 = local read "Actual Field (T)"() -> (w388:dbl)
                  n153 = local read "Min Field (T)"() -> (w387:dbl)
                  n154 = local read "Stepping Mode"() -> (w385:bool)
                  n155 = local read "Max Field (T)"() -> (w393:dbl)
                  n156 = case shown="True" w385 {
                    tunnel: [w394 w395] -> w386
                    frame False {
                      n157 = local read "Read?"() -> (w394:bool)
                    }
                    frame True {
                      n158 = local read "Ready2Step"() -> (w395:bool)
                    }
                  }
                  n159 = Greater Or Equal?(x=w387, y=w388) -> (x >= y?=w390:bool)
                  n160 = Compound Arithmetic op=AND(w390, w386) -> (w389:bool)
                  n161 = case shown="False" w389 {
                    tunnel: [w398 w437] -> w391
                    tunnel: w393 -> [w396 w436]
                    tunnel: w387 -> [_ w435]
                    tunnel: w388 -> [_ w433]
                    tunnel: w392 -> [w399 w432]
                    frame True {
                      # "Ramp Up"
                      n162 = case shown="False" "First?" {
                        tunnel: [TRUE ("Save") FALSE ("Save")] -> w402
                        tunnel: [w424 w428] -> w401
                        frame False {
                          n163 = local read "Counter"() -> (w427:i8)
                          n164 = local write "Actual Polarization"(0.0 ("Actual Polarization")) -> ()
                          n165 = Increment(x=w427) -> (x+1=w424:i8)
                          n166 = local write "Counter"(w424) -> ()
                        }
                        frame True {
                          n167 = local read "Counter"() -> (w428:i8)
                          n168 = local write "First?"(FALSE ("First?")) -> ()
                        }
                      }
                      "Reset" <- w402
                      n169 = local write "Read?"(FALSE ("Read?")) -> ()
                      n170 = local read "Record ALL"() -> (w397:bool)
                      n171 = case shown="True" w397 {
                        tunnel: w401 -> [_ w409]
                        tunnel: [FALSE w407] -> w400
                        frame False {
                        }
                        frame True {
                          n172 = Greater?(x=w409, y="Max Countl") -> (0:w407:bool)
                        }
                      }
                      n173 = case shown="False" w400 {
                        tunnel: w399 -> [w416 w423]
                        tunnel: [w415 w423] -> w398
                        tunnel: w396 -> [w414 _]
                        frame False {
                          n174 = local read "Magnet"() -> (w411:bool)
                          n175 = Not(x="Stepping Mode") -> (.not. x?=w412:bool)
                          n176 = And(x=w412, y=w411) -> (x .and. y?=w410:bool)
                          n177 = case shown="True" w410 {
                            tunnel: w416 -> [w417 w420]
                            tunnel: [w417 w419] -> w415
                            tunnel: w414 -> [_ w418]
                            frame False {
                            }
                            frame True {
                              n178 = call "Set_B.vi"("error in (no error)"=w420, "address string"="25", "Set Field (T)"=w418) -> ("error out"=w419:errorcluster)  [unwired: 8 in]
                            }
                          }
                          "Target Field" <- w414
                        }
                        frame True {
                          "New" <- TRUE
                        }
                      }
                      "Up/Down" <- FALSE ("Up/Down")
                    }
                    frame False {
                      n179 = Less Or Equal?(x=w436, y=w433) -> (x <= y?=w434:bool)
                      n180 = case shown="True" w434 {
                        tunnel: [w438 w445] -> w437
                        tunnel: w435 -> [_ w443]
                        tunnel: w432 -> [w438 w446]
                        frame False {
                        }
                        frame True {
                          # "Resetting at the end of every cycle"
                          # "Ramp Dn"
                          n181 = local write "Up/Down"(TRUE ("Up/Down")) -> ()
                          n182 = local read "Stepping Mode"() -> (w442:bool)
                          n183 = local read "Magnet"() -> (w441:bool)
                          n184 = local write "Target Field"(w443) -> ()
                          n185 = Not(x=w442) -> (.not. x?=w439:bool)
                          n186 = local write "Reset"(TRUE ("Reset")) -> ()
                          n187 = And(x=w441, y=w439) -> (x .and. y?=w440:bool)
                          n188 = case shown="False" w440 {
                            tunnel: w446 -> [w448 w451]
                            tunnel: [w448 w450] -> w445
                            tunnel: w443 -> [_ w449]
                            frame False {
                            }
                            frame True {
                              n189 = call "Set_B.vi"("error in (no error)"=w451, "address string"="25", "Set Field (T)"=w449) -> ("error out"=w450:errorcluster)  [unwired: 8 in]
                            }
                          }
                        }
                      }
                      n190 = local write "Read?"(FALSE ("Read?")) -> ()
                    }
                  }
                }
                frame True {
                  n191 = local read "Setpoint Temperature (K)"() -> (w455:dbl)
                  n192 = local read "Min Temperature (K)"() -> (w454:dbl)
                  n193 = local read "Read?"() -> (w460:bool)
                  n194 = local read "Max temperature (K)"() -> (w453:dbl)
                  n195 = Equal?(x=w455, y=w454) -> (x = y?=w458:bool)
                  n196 = And(x=w458, y=w460) -> (x .and. y?=w459:bool)
                  n197 = case shown="False" w459 {
                    tunnel: [w462 w479] -> w456
                    tunnel: w453 -> [w461 w478]
                    tunnel: w454 -> [_ w477]
                    tunnel: w455 -> [_ w475]
                    tunnel: w457 -> [w463 w474]
                    frame True {
                      # "Ramp Up"
                      n198 = local read "First?"() -> (w469:bool)
                      n199 = case shown="False" w469 {
                        frame False {
                          n200 = local read "Counter"() -> (w472:i8)
                          n201 = Increment(x=w472) -> (x+1=w471:i8)
                          n202 = local write "Counter"(w471) -> ()
                        }
                        frame True {
                        }
                      }
                      n203 = local write "Read?"(FALSE ("Read?")) -> ()
                      n204 = Number To Fractional String(number=w461, precision (6)=i16 3) -> (F-format string=w466:string)  [unwired: 2 in]
                      n205 = local read "Lake Shore"() -> (w464:refnum<visa-resource-name>)
                      n206 = Concatenate Strings("SETP 1," ("write buffer"), w466) -> (w468:string)
                      n207 = VISA Write(VISA resource name=w464, write buffer=w468, error in (no error)=w463) -> (error out=w462:errorcluster)  [unwired: 2 out]
                    }
                    frame False {
                      n208 = Equal?(x=w478, y=w475) -> (x = y?=w476:bool)
                      n209 = case shown="True" w476 {
                        tunnel: [w480 w483] -> w479
                        tunnel: w477 -> [_ w482]
                        tunnel: w474 -> [w480 w484]
                        frame False {
                        }
                        frame True {
                          # "Ramp Dn"
                          n210 = local write "Up/Down"(TRUE ("Up/Down")) -> ()
                          n211 = Number To Fractional String(number=w482, precision (6)=i16 3) -> (F-format string=w486:string)  [unwired: 2 in]
                          n212 = local read "Lake Shore"() -> (w481:refnum<visa-resource-name>)
                          n213 = Concatenate Strings("SETP 1," ("write buffer"), w486) -> (w488:string)
                          n214 = VISA Write(VISA resource name=w481, write buffer=w488, error in (no error)=w484) -> (error out=w483:errorcluster)  [unwired: 2 out]
                        }
                      }
                      n215 = local write "Read?"(FALSE ("Read?")) -> ()
                    }
                  }
                }
              }
              n216 = local read "Magnet"() -> (w368:bool)
              n217 = case shown="True" w368 {
                tunnel: [Mode."StepDelta" ("Enum") w382] -> w370
                frame False {
                }
                frame True {
                  n218 = local read "Stepping Mode"() -> (w381:bool)
                  n219 = case shown="True" w381 {
                    tunnel: [Mode."Plot" ("Enum") Mode."StepDelta" ("Enum")] -> w382
                    frame False {
                    }
                    frame True {
                    }
                  }
                }
              }
            }
            frame "StepDelta" {
              n220 = local read "Stepping Mode"() -> (w492:bool)
              n221 = case shown="True" w492 {
                tunnel: w494 -> [w503 w564]
                tunnel: [w502 w555] -> w493
                tunnel: w491 -> [_ w557]
                tunnel: [w501 w558] -> w490
                frame False {
                  n222 = flat-sequence {
                    tunnel: w503 -> [w512]
                    tunnel: [w511] -> w502
                    tunnel: [Mode."Plot" ("Enum")] -> w501
                    frame #0 {
                      # "Check if it is time to step Field"
                      n223 = local read "Sweep Rate (T/min)"() -> (w513:dbl)
                      n224 = local read "B/V (T/V)"() -> (w505:dbl)
                      n225 = local read "Time Lag"() -> (w509:dbl)
                      n226 = xnode "Sweep Delay"("SweepRate"=w513, "Resolution"=0.001 ("Voltage Step (V)"), "BpV"=w505) -> ("Result"=w510:dbl)  [unwired: 1 in, 1 out]
                      n227 = Divide(x=w509, y=w510) -> (x/y=w507:dbl)
                      n228 = Multiply(x=0.001 ("y"), y=w507) -> (x*y=w506:dbl)
                      "deltaUaux" <- w506
                      n229 = stacked-sequence {
                        tunnel: w512 -> [_ w537]
                        tunnel: [_ w536] -> w511
                        tunnel: w506 -> [w515 _]
                        frame #0 {
                          n230 = local read "Actual Voltage (V)"() -> (w520:dbl)
                          n231 = local read "Up/Down"() -> (w521:bool)
                          n232 = Add(x=w520, y=w515) -> (x+y=w517:dbl)
                          n233 = Subtract(x=w520, y=w515) -> (x-y=w516:dbl)
                          n234 = Select(t=w516, s=w521, f=w517) -> (s? t:f=w519:dbl)
                          "Actual Voltage (V)" <- w519
                          n235 = local read "V/I (Ohm)"() -> (w522:dbl)
                          n236 = local read "B/V (T/V)"() -> (w523:dbl)
                          n237 = xnode "AUXtoB"("BpV"=w523, "Rm"=w522, "Aux"=w519) -> ("Result"=w518:dbl)  [unwired: 1 in, 1 out]
                          n238 = local write "Actual Field (T)"(w518) -> ()
                        }
                        frame #1 {
                          n239 = local read "Actual Voltage (V)"() -> (w542:dbl)
                          n240 = local read "Lock_in_Amplifier"() -> (w538:refnum<visa-resource-name>)
                          n241 = Format Into String(w542) -> (resulting string=w541:string)  [unwired: 3 in, 1 out]
                          n242 = Concatenate Strings("AUXV 1,", w541) -> (w539:string)
                          n243 = VISA Write(VISA resource name=w538, write buffer=w539, error in (no error)=w537) -> (error out=w536:errorcluster)  [unwired: 2 out]
                        }
                      }
                    }
                  }
                }
                frame True {
                  n244 = case shown="True" "Ready2Step" {
                    tunnel: w564 -> [w565 w571]
                    tunnel: [w565 w570] -> w556
                    frame False {
                    }
                    frame True {
                      n245 = local read "Actual Field (T)"() -> (w575:dbl)
                      n246 = local read "Up/Down"() -> (w568:bool)
                      n247 = Add(x=w575, y="Field Step (T)") -> (x+y=w567:dbl)
                      n248 = Subtract(x=w575, y="Field Step (T)") -> (x-y=w566:dbl)
                      n249 = Select(t=w566, s=w568, f=w567) -> (s? t:f=w573:dbl)
                      n250 = call "Set_B.vi"("error in (no error)"=w571, "address string"="25", "Set Field (T)"=w573) -> ("error out"=w570:errorcluster)  [unwired: 8 in]
                      n251 = local write "Ready2Step"(FALSE ("Ready2Step")) -> ()
                    }
                  }
                  n252 = local read "Last2"() -> (w561:dbl)
                  n253 = Quotient & Remainder(x=w557, y="Window (s)") -> (floor(x/y)=w562:dbl)  [unwired: 1 out]
                  "Actual2" <- w562
                  n254 = Greater?(x=w562, y=w561) -> (0:w560:bool)
                  n255 = case shown="True" w560 {
                    tunnel: w562 -> [_ w583]
                    tunnel: [Mode."Plot" ("Enum") w582] -> w558
                    tunnel: w556 -> [w576 w580]
                    tunnel: [w576 w580] -> w555
                    frame False {
                      n256 = local read "Actual Current (pA)"() -> (→"I(t)":dbl)
                      n257 = local read "Actual Field (T)"() -> (→"B(t)":dbl)
                    }
                    frame True {
                      n258 = case shown="True" "ReOffset" {
                        tunnel: [Mode."Plot" ("Enum") Mode."Offset" ("Enum")] -> w582
                        frame False {
                          n259 = local write "Ready2Step"(TRUE ("Ready2Step")) -> ()
                        }
                        frame True {
                          n260 = local read "Dwell Time (s)"() -> (w590:dbl)
                          n261 = local read "Time Lag"() -> (w589:dbl)
                          n262 = local write "Offset?"(FALSE ("Offset?")) -> ()
                          n263 = local write "Offset array"(dbl[] []) -> ()
                          n264 = Divide(x=w590, y=w589) -> (x/y=w588:dbl)
                          n265 = local write "Count"(w588) -> ()
                        }
                      }
                      "Last2" <- w583
                    }
                  }
                }
              }
            }
            frame "Plot" {
              # "dI"
              n266 = local read "No pol"() -> (w592:bool)
              n267 = local read "Actual Current (pA)"() -> (w594:dbl)
              n268 = local read "P(uC/mm^2)"() -> (w593:dbl[])
              n269 = local read "Time Lag"() -> (w606:dbl)
              n270 = Multiply(x=w594, y=w606) -> (x*y=w598:dbl)
              n271 = Divide(x=w598, y="Sample area (mm^2)") -> (x/y=w597:dbl)
              n272 = case shown="True" w592 {
                tunnel: w597 -> [w613 _]
                tunnel: [w612 w615] -> w596
                frame False {
                  n273 = local read "Actual Polarization"() -> (w611:dbl)
                  n274 = Add(x=w613, y=w611) -> (x+y=w612:dbl)
                }
                frame True {
                  n275 = local read "Actual Polarization"() -> (w617:dbl)
                  n276 = local write "No pol"(FALSE ("No pol")) -> ()
                  n277 = Add(x=w617, y=0.0) -> (x+y=w615:dbl)
                }
              }
              "Actual Polarization" <- w596
              n278 = local read "Temp/Magnetic Field"() -> (w607:bool)
              n279 = Build Array (concatenate)(w593, w596) -> (→"P(uC/mm^2)":dbl[])
              n280 = case shown="False" w607 {
                tunnel: w604 -> [_ w674]
                tunnel: w601 -> [_ w656]
                tunnel: w596 -> [w621 w657]
                frame False {
                  # "Magnetic Field plotting"
                  n281 = local read "Up/Down"() -> (w626:bool)
                  n282 = case shown="True" w626 {
                    frame True {
                      # "Down"
                      n283 = local read "I(B) 3"() -> (w636:cluster{dbl[], dbl[]}[])
                      n284 = local read "I(B) 3"() -> (w640:cluster{dbl[], dbl[]}[])
                      n285 = Index Array(array=w636, index=1) -> (element=w634:cluster{dbl[], dbl[]})
                      n286 = Unbundle(w634) -> (w633:dbl[], w632:dbl[])
                      n287 = Index Array(array=w640, index=i8 0 ("t")) -> (element=w637:cluster{dbl[], dbl[]})
                      n288 = local read "Actual Current (pA)"() -> (w627:dbl)
                      n289 = local read "Actual B Field (T)"() -> (w629:dbl)
                      n290 = Build Array (concatenate)(w633, w629) -> (w631:dbl[])
                      n291 = Build Array (concatenate)(w632, w627) -> (w630:dbl[])
                      n292 = Bundle(w631, w630) -> (w628:cluster{dbl[], dbl[]})  [unwired: 1 in]
                      n293 = Build Array(w637, w628) -> (w638:cluster{dbl[], dbl[]}[])
                      n294 = local write "I(B) 3"(w638) -> ()
                    }
                    frame False {
                      # "Up"
                      n295 = local read "I(B) 3"() -> (w652:cluster{dbl[], dbl[]}[])
                      n296 = local read "I(B) 3"() -> (w654:cluster{dbl[], dbl[]}[])
                      n297 = Index Array(array=w652, index=0) -> (element=w650:cluster{dbl[], dbl[]})
                      n298 = Unbundle(w650) -> (w649:dbl[], w648:dbl[])
                      n299 = Index Array(array=w654, index=i8 1 ("t")) -> (element=w643:cluster{dbl[], dbl[]})
                      n300 = local read "Actual B Field (T)"() -> (w644:dbl)
                      n301 = Build Array (concatenate)(w649, w644) -> (w647:dbl[])
                      n302 = local read "Actual Current (pA)"() -> (w641:dbl)
                      n303 = Build Array (concatenate)(w648, w641) -> (w646:dbl[])
                      n304 = Bundle(w647, w646) -> (w645:cluster{dbl[], dbl[]})  [unwired: 1 in]
                      n305 = Build Array(w645, w643) -> (w642:cluster{dbl[], dbl[]}[])
                      n306 = local write "I(B) 3"(w642) -> ()
                    }
                  }
                  n307 = local read "Actual B Field (T)"() -> (w623:dbl)
                  n308 = local read "P(B)"() -> (w625:cluster{"yi":dbl[], dbl[]})
                  n309 = Unbundle(w625) -> ("yi"=w624:dbl[], w622:dbl[])
                  n310 = Build Array (concatenate)(w624, w623) -> (w620:dbl[])
                  n311 = Build Array (concatenate)(w622, w621) -> (w619:dbl[])
                  n312 = Bundle(w620, w619) -> (→"P(B)":cluster{dbl[], dbl[]})  [unwired: 1 in]
                }
                frame True {
                  # "Temperature plotting"
                  n313 = Quotient & Remainder(x=w674, y="Save Period") -> (x-y*floor(x/y)=w655:dbl)  [unwired: 1 out]
                  n314 = Greater?(x=w656, y=w655) -> (0:w672:bool)
                  n315 = local read "Actual Temperature (K)"() -> (w659:dbl)
                  n316 = local read "Actual Current (pA)"() -> (w665:dbl)
                  n317 = local read "P(T)"() -> (w661:cluster{"yi":dbl[], dbl[]})
                  n318 = local read "I(T)"() -> (w671:cluster{dbl[], dbl[]})
                  n319 = case shown="True" w672 {
                    frame False {
                    }
                    frame True {
                      n320 = local write "Reset"(TRUE) -> ()
                    }
                  }
                  n321 = Unbundle(w661) -> ("yi"=w662:dbl[], w658:dbl[])
                  n322 = Unbundle(w671) -> (w669:dbl[], w668:dbl[])
                  n323 = Build Array (concatenate)(w662, w659) -> (w663:dbl[])
                  n324 = Build Array (concatenate)(w658, w657) -> (w664:dbl[])
                  n325 = Build Array (concatenate)(w669, w659) -> (w667:dbl[])
                  n326 = Build Array (concatenate)(w668, w665) -> (w666:dbl[])
                  n327 = Bundle(w667, w666) -> (→"I(T)":cluster{dbl[], dbl[]})  [unwired: 1 in]
                  n328 = Bundle(w663, w664) -> (→"P(T)":cluster{dbl[], dbl[]})  [unwired: 1 in]
                }
              }
            }
            frame "Save" {
              n329 = local read "Reset"() -> (w676:bool)
              n330 = case shown="True" w676 {
                tunnel: w681 -> [w698 w700]
                tunnel: [w698 w703] -> w686
                tunnel: w680 -> [w697 w701]
                tunnel: [w697 w703] -> w685
                tunnel: w682 -> [w696 w702]
                tunnel: [w696 w703] -> w684
                tunnel: [w695 w703] -> w683
                tunnel: w679 -> [w695 w699]
                frame False {
                }
                frame True {
                  n331 = stacked-sequence {
                    tunnel: [_ _ w755] -> w703
                    tunnel: w702 -> [_ w744 _]
                    tunnel: w701 -> [w730 w742 _]
                    tunnel: w700 -> [w731 w743 _]
                    tunnel: w699 -> [w720 w740 _]
                    frame #0 {
                      n332 = local read "B array"() -> (w714:dbl[])
                      n333 = local read "Counter"() -> (w729:i8)
                      n334 = local read "Averaged I(B)"() -> (w704:dbl[][])
                      n335 = local read "Up/Down"() -> (w732:bool)
                      n336 = local read "Sample area (mm^2)"() -> (w710:dbl)
                      n337 = call "Average_IBP_curves_baseline.vi"("I in"=w730, "Averaged P(B) In"="Averaged P(B)", "Counter"=w729, "B0"="Threshold B (T)", "Averaged I(B) In"=w704, "t in"=w720, "B in"=w731, "Averaged dt in"="Averaged dt", "Up/Down"=w732, "Sample area(mm^2)"=w710, "B array"=w714) -> ("Averaged I(B) out"=→"Averaged I(B)":dbl[][], "Averaged dt Out"=w717:dbl[][], "Averaged P(B) Out"=w706:dbl[][], "BaselineSubtracted I(B)"=w705:dbl[][])  [unwired: 1 in]
                      n338 = Index Array(array=w706, index (row)=0 ("disabled index (col)")) -> (element=w715:dbl[])  [unwired: 1 in]
                      n339 = Index Array(array=w706, index (row)=1 ("disabled index (col)")) -> (element=w716:dbl[])  [unwired: 1 in]
                      n340 = Index Array(array=w705, index (row)=0 ("disabled index (col)")) -> (element=w722:dbl[])  [unwired: 1 in]
                      n341 = Index Array(array=w705, index (row)=1 ("disabled index (col)")) -> (element=w721:dbl[])  [unwired: 1 in]
                      n342 = local write "Averaged dt"(w717) -> ()
                      n343 = Bundle("B array"=w714, "Averaged P(B) Out"=w715) -> (w713:T7)  [unwired: 1 in]
                      n344 = Bundle("B array"=w714, "Averaged P(B) Out"=w716) -> (w712:T7)  [unwired: 1 in]
                      n345 = local write "Averaged P(B)"(w706) -> ()
                      n346 = Bundle("B array"=w714, "BaselineSubtracted I(B)"=w722) -> (w728:T8)  [unwired: 1 in]
                      n347 = Bundle("B array"=w714, "BaselineSubtracted I(B)"=w721) -> (w727:T8)  [unwired: 1 in]
                      n348 = Build Array(w713, w712) -> (→"P(B) /Averaged/":T9)
                      n349 = Build Array(w728, w727) -> (→"I(B) /Averaged/":T10)
                    }
                    frame #1 {
                      # "Save and Reset"
                      n350 = local read "Temp/Magnetic Field"() -> (w733:bool)
                      n351 = local read "Measurement File"() -> (w735:path)
                      n352 = local read "P(uC/mm^2)"() -> (w741:dbl[])
                      n353 = Build Array(w744, w743, w742, w740, w741) -> (w734:dbl[][])
                      n354 = case shown="False" w733 {
                        tunnel: w735 -> [_ _]
                        tunnel: w734 -> [w749 _]
                        frame False {
                          n355 = local read "Up/Down"() -> (w747:bool)
                          n356 = case shown="True" w747 {
                            tunnel: [w752 w753] -> w746
                            frame False {
                              n357 = local read "Measurement File_dn"() -> (w752:path)
                            }
                            frame True {
                              n358 = local read "Measurement File_up"() -> (w753:path)
                            }
                          }
                          n359 = call-poly <vilib>:"Write Delimited Spreadsheet.vi"("file path (dialog if empty)"=w746, "format (%.3f)"="%.5g", "2D data"=w749, "append to file? (F)"=TRUE ("transpose? (F)"), "transpose? (F)"=FALSE ("append to file? (F)")) -> ()  [unwired: 9 in, 2 out]
                        }
                        frame True {
                        }
                      }
                      n360 = case shown="False" "Reset IB?" {
                        frame False {
                        }
                        frame True {
                          n361 = local read "Up/Down"() -> (w754:bool)
                          n362 = case shown="False" w754 {
                            frame False {
                              n363 = invoke on="I(B) 3" class="XYGraph (strict)" method="Reinit To Default"() -> ()  [unwired: 3 in, 3 out]
                            }
                            frame True {
                            }
                          }
                        }
                      }
                      n364 = call-poly <vilib>:"Write Delimited Spreadsheet.vi"("file path (dialog if empty)"=w735, "format (%.3f)"="%.5g", "2D data"=w734, "append to file? (F)"=TRUE, "transpose? (F)"=TRUE) -> ()  [unwired: 9 in, 2 out]
                      n365 = local write "Reset"(FALSE ("Save")) -> ()
                    }
                    frame #2 {
                      w755 = dbl[] []
                      n366 = local write "P(uC/mm^2)"(w755) -> ()
                    }
                  }
                }
              }
              n367 = local read "New"() -> (w678:bool)
              n368 = case shown="False" w678 {
                tunnel: [Mode."Return" ("Enum") Mode."New" ("Enum")] -> w690
                tunnel: [TRUE FALSE] -> w677
                frame False {
                }
                frame True {
                }
              }
            }
            frame "New" {
              n369 = stacked-sequence {
                seq-local: [_ _ _ _ w857 _ _] -> [_ _ _ _ _ w866 _]
                seq-local: [_ _ w811 _ _ _ _] -> [_ _ _ _ w856 _ _]
                tunnel: T6 {"Com Port"=1, "ISOBUS Address"=0, "GPIB Address"=25, "Communication"=enum."GPIB"} ("Address") -> [_ _ w810 w851 _ _ _]
                tunnel: w758 -> [_ _ w812 _ _ w867 _]
                tunnel: [_ _ _ _ _ w869 _] -> w757
                tunnel: w756 -> [_ w791 _ _ _ _ _]
                frame #0 {
                  w784 = 1 ("index (row)")
                  w783 = 0 ("index (row)")
                  # "Save averages"
                  n370 = local read "Measurement File_average"() -> (w771:path)
                  n371 = local read "Averaged P(B)"() -> (w782:dbl[][])
                  n372 = local read "Averaged dt"() -> (w780:dbl[][])
                  n373 = local read "I(B) /Averaged/"() -> (w772:cluster{"B array":dbl[], dbl[]}[])
                  n374 = Index Array(array=w780, index (row)=w783) -> (element=w781:dbl[])  [unwired: 1 in]
                  n375 = Index Array(array=w780, index (row)=w784) -> (element=w788:dbl[])  [unwired: 1 in]
                  n376 = Index Array(array=w772, index=1) -> (element=w776:cluster{"B array":dbl[], dbl[]})
                  n377 = Index Array(array=w772, index=0) -> (element=w775:cluster{"B array":dbl[], dbl[]})
                  n378 = Unbundle(w776) -> ("B array"=w786:dbl[], w787:dbl[])
                  n379 = Unbundle(w775) -> ("B array"=w777:dbl[], w778:dbl[])
                  n380 = Index Array(array=w782, index (row)=w783) -> (element=w785:dbl[])  [unwired: 1 in]
                  n381 = Index Array(array=w782, index (row)=w784) -> (element=w789:dbl[])  [unwired: 1 in]
                  n382 = Build Array(w777, w778, w781, w785, w786, w787, w788, w789) -> (w779:dbl[][])
                  n383 = call-poly <vilib>:"Write Delimited Spreadsheet.vi"("file path (dialog if empty)"=w771, "format (%.3f)"="%.5g", "2D data"=w779, "append to file? (F)"=TRUE ("transpose? (F)"), "transpose? (F)"=TRUE ("append to file? (F)")) -> ()  [unwired: 9 in, 2 out]
                }
                frame #1 {
                  w797 = dbl[] []
                  w806 = dbl[] []
                  # "Reset Flags"
                  n384 = Get Date/Time In Seconds() -> (seconds since 1Jan1904=w807:timestamp)
                  n385 = local write "Up/Down"(TRUE ("Up/Down")) -> ()
                  n386 = local write "First?"(TRUE ("First?")) -> ()
                  n387 = local write "Offset?"(FALSE ("Offset?")) -> ()
                  n388 = local write "New"(FALSE ("New")) -> ()
                  n389 = local write "P(uC/mm^2)"(w806) -> ()
                  n390 = local write "Start time"(w807) -> ()
                  n391 = local write "Offset array"(w806) -> ()
                  n392 = local write "Actual Polarization"(0.0 ("Actual Polarization")) -> ()
                  n393 = local write "Up/Down"(TRUE ("Up/Down")) -> ()
                  n394 = local write "Reset"(FALSE ("Reset")) -> ()
                  n395 = local read "B array"() -> (w800:dbl[])
                  n396 = local write "Counter"(i8 0 ("Counter")) -> ()
                  n397 = invoke on="P(B)" class="XYGraph (strict)" method="Reinit To Default"() -> ()  [unwired: 3 in, 3 out]
                  n398 = invoke on="I(B) 3" class="XYGraph (strict)" method="Reinit To Default"() -> ()  [unwired: 3 in, 3 out]
                  n399 = Multiply(x=w800, y=0.0) -> (x*y=w801:dbl[])
                  n400 = Build Array(w797, w797) -> (w805:dbl[][])
                  n401 = Bundle("B array"=w800, w801) -> (w802:cluster{"B array":dbl[], dbl[]})  [unwired: 1 in]
                  n402 = local write "Averaged I(B)"(w805) -> ()
                  n403 = Build Array(w802, w802) -> (w803:cluster{"B array":dbl[], dbl[]}[])
                  n404 = local write "I(B) /Averaged/"(w803) -> ()
                  n405 = local write "Measuring"(FALSE ("Measuring")) -> ()
                  n406 = Flush Queue(queue=w791) -> (remaining elements=→"remaining elements 2":T1)  [unwired: 1 in, 2 out]
                }
                frame #2 {
                  # "Step"
                  n407 = local read "Sweep Rate Array"() -> (w816:dbl[])
                  n408 = local read "j"() -> (w817:i32)
                  n409 = Increment(x=w817) -> (x+1=w813:i32)
                  n410 = Array Size(array=w816) -> (size(s)=w815:i32)
                  n411 = Less?(x=w813, y=w815) -> (x < y?=w814:bool)
                  "Step Rate" <- w814
                  n412 = case shown="True" w814 {
                    tunnel: w813 -> [_ w844]
                    tunnel: w812 -> [w820 w843]
                    tunnel: [w819 w843] -> w811
                    tunnel: w810 -> [w818 _]
                    frame False {
                      # "Step Temp?"
                      n413 = local read "Temperature Array"() -> (w824:dbl[])
                      n414 = local read "i"() -> (w825:i32)
                      n415 = Increment(x=w825) -> (x+1=w822:i32)
                      n416 = local write "j"(0 ("f")) -> ()
                      n417 = Array Size(array=w824) -> (size(s)=w823:i32)
                      n418 = Less?(x=w822, y=w823) -> (x < y?=w821:bool)
                      "Step Temp" <- w821
                      n419 = case shown="False" w821 {
                        tunnel: w822 -> [_ w842]
                        tunnel: w820 -> [w830 w841]
                        tunnel: [w829 w841] -> w819
                        tunnel: w818 -> [w828 _]
                        frame False {
                          # "Heater OFF"
                          # "Finished"
                          n420 = local write "i"(0 ("i")) -> ()
                          n421 = stacked-sequence {
                            tunnel: w830 -> [w834 _ _]
                            tunnel: [w833 _ _] -> w829
                            tunnel: w828 -> [_ w838 w839]
                            frame #0 {
                              n422 = local read "Lake Shore"() -> (w835:refnum<visa-resource-name>)
                              n423 = VISA Write(VISA resource name=w835, write buffer="RANGE,1,0", error in (no error)=w834) -> (error out=w833:errorcluster)  [unwired: 2 out]
                            }
                            frame #1 {
                              n424 = call "ips_switchHeaterOff.vi"("Instrument address"=w838, "Rate"=2.0) -> ()  [unwired: 1 out]
                            }
                            frame #2 {
                              n425 = call "GPIB - BusCommand.vi"("Command"="H0", "Address"=w839) -> ()  [unwired: 2 out]
                            }
                          }
                          n426 = local write "Record ALL"(FALSE ("Record ALL")) -> ()
                          "Finished" <- TRUE
                        }
                        frame True {
                          n427 = local write "i"(w842) -> ()
                        }
                      }
                    }
                    frame True {
                      n428 = local write "j"(w844) -> ()
                    }
                  }
                }
                frame #3 {
                  # "Set rates"
                  n429 = local read "Sweep Rate Array"() -> (w850:dbl[])
                  n430 = local read "j"() -> (w849:i32)
                  n431 = local read "j"() -> (w847:i32)
                  n432 = Index Array(array=w850, index=w849) -> (element=w848:dbl)
                  n433 = Number To Fractional String(number=w848, precision (6)=i16 3) -> (F-format string=w854:string)  [unwired: 2 in]
                  n434 = Index Array(array="Max count array", index=w847) -> (element=w845:i32)
                  n435 = local write "Max Countl"(w845) -> ()
                  n436 = Concatenate Strings("T" ("format string"), w854) -> (w855:string)
                  n437 = call "GPIB - BusCommand.vi"("Command"=w855, "Address"=w851) -> ()  [unwired: 2 out]
                  n438 = local write "Sweep Rate (T/min)"(w848) -> ()
                }
                frame #4 {
                  # "Set temperature"
                  n439 = local read "Temperature Array"() -> (w860:dbl[])
                  n440 = local read "i"() -> (w859:i32)
                  n441 = Index Array(array=w860, index=w859) -> (element=w858:dbl)
                  n442 = local read "Lake Shore"() -> (w862:refnum<visa-resource-name>)
                  n443 = Number To Fractional String(number=w858, precision (6)=i16 3) -> (F-format string=w863:string)  [unwired: 2 in]
                  n444 = Concatenate Strings("SETP 1," ("write buffer"), w863) -> (w865:string)
                  n445 = VISA Write(VISA resource name=w862, write buffer=w865, error in (no error)=w856) -> (error out=w857:errorcluster)  [unwired: 2 out]
                }
                frame #5 {
                  n446 = local read "Finished"() -> (w868:bool)
                  n447 = case shown="False" w868 {
                    tunnel: [w882 w919] -> w869
                    tunnel: w867 -> [_ _]
                    tunnel: w866 -> [w879 w919]
                    frame False {
                      w877 = "_" ("string")
                      # "Wait, create Files"
                      n448 = local read "Temperature Array"() -> (w909:dbl[])
                      n449 = local read "Sweep Rate Array"() -> (w905:dbl[])
                      n450 = local read "i"() -> (w908:i32)
                      n451 = local read "j"() -> (w906:i32)
                      n452 = Index Array(array=w909, index=w908) -> (element=w907:dbl)
                      n453 = Index Array(array=w905, index=w906) -> (element=w874:dbl)
                      n454 = Round Toward -Infinity(1:w874) -> (0:w875:dbl)
                      n455 = Number To Fractional String(use system decimal point (T)=TRUE, number=w907, precision (6)=i16 1) -> (F-format string=w910:string)  [unwired: 1 in]
                      n456 = Subtract(x=w874, y=w875) -> (x-y=w876:dbl)
                      n457 = Equal To 0?(x=w876) -> (x = 0?=w873:bool)
                      n458 = Select(t=i16 0 ("precision (6)"), s=w873, f=i16 2 ("precision (6)")) -> (s? t:f=w870:i16)
                      n459 = Number To Fractional String(use system decimal point (T)=TRUE, number=w874, precision (6)=w870) -> (F-format string=w878:string)  [unwired: 1 in]
                      n460 = Concatenate Strings("Directory", "\\" ("string"), "FileName", w877, w910, "K" ("string"), w877, w878, "Tpm" ("string")) -> (w899:string)
                      n461 = Search and Replace String(replace all?=TRUE ("replace all? (F)"), input string=w899, search string=".", replace string="p" ("substring (\"\")"), error in=w879) -> (result string=w894:string, error out=w889:errorcluster)  [unwired: 3 in, 2 out]
                      n462 = local write "Step Rate"(FALSE ("Step Rate")) -> ()
                      n463 = Concatenate Strings(w894, ".txt" ("string")) -> (w893:string)
                      n464 = local read "Step Temp"() -> (w883:bool)
                      n465 = String To Path(string=w893) -> (path=w892:path)
                      n466 = Open/Create/Replace File(file path (use dialog)=w892, error in=w889, operation (0:open)=T5."open or create") -> (refnum out=w881:refnum<file>, error out=w882:errorcluster)  [unwired: 3 in, 1 out]
                      n467 = local write "refnum out"(w881) -> ()
                      n468 = Refnum to Path(1:w881) -> (0:w884:path)
                      n469 = call "Create_sweep_files.vi"("Measurement File"=w884) -> ("Path 3"=w887:path, "Path 2"=w886:path, "Path"=w885:path)  [unwired: 8 in]
                      n470 = local write "Measurement File"(w884) -> ()
                      n471 = case shown="True" w883 {
                        frame False {
                        }
                        frame True {
                          n472 = Get Date/Time In Seconds() -> (seconds since 1Jan1904=w912:timestamp)
                          n473 = local write "Step Temp"(FALSE ("Step Temp")) -> ()
                          n474 = while {
                            tunnel: w912 -> [w917]
                            stop <- w914 stop-if-true
                            n475 = Get Date/Time In Seconds() -> (seconds since 1Jan1904=w918:timestamp)
                            n476 = Subtract(x=w918, y=w917) -> (x-y=w916:dbl)
                            "Wait (s)" <- w916
                            n477 = Greater Or Equal?(x=w916, y="secs to wait") -> (x >= y?=w914:bool)
                          }
                        }
                      }
                      n478 = local write "Measurement File_dn"(w887) -> ()
                      n479 = local write "Measurement File_average"(w885) -> ()
                      n480 = local write "Measurement File_up"(w886) -> ()
                    }
                    frame True {
                    }
                  }
                }
                frame #6 {
                  n481 = local read "Finished"() -> (w920:bool)
                  n482 = case shown="True" w920 {
                    frame False {
                      n483 = local write "Measuring"(TRUE ("Measuring")) -> ()
                    }
                    frame True {
                      n484 = local write "Measure /Pause"(FALSE ("Measure /Pause")) -> ()
                    }
                  }
                }
              }
            }
            frame "Return" {
            }
          }
        }
      }
      frame Error {
        # "Return true for any case which should stop the loop."
      }
    }
  }
  n485 = case shown="True" w54 {
    frame False {
    }
    frame True {
      n486 = local read "B array"() -> (w943:dbl[])
      n487 = invoke on="P(T)" class="XYGraph (strict)" method="Reinit To Default"() -> ()  [unwired: 3 in, 3 out]
      n488 = invoke on="I(T)" class="XYGraph (strict)" method="Reinit To Default"() -> ()  [unwired: 3 in, 3 out]
      n489 = invoke on="P(B)" class="XYGraph (strict)" method="Reinit To Default"() -> ()  [unwired: 3 in, 3 out]
      n490 = invoke on="I(B) 3" class="XYGraph (strict)" method="Reinit To Default"() -> ()  [unwired: 3 in, 3 out]
      n491 = Multiply(x=w943, y=0.0) -> (x*y=w942:dbl[])
      n492 = Bundle("B array"=w943, w942) -> (w941:cluster{"B array":dbl[], dbl[]})  [unwired: 1 in]
      n493 = Build Array(w941, w941) -> (w940:cluster{"B array":dbl[], dbl[]}[])
      n494 = local write "I(B) /Averaged/"(w940) -> ()
      n495 = invoke on="P(B) /Averaged/" class="XYGraph (strict)" method="Reinit To Default"() -> ()  [unwired: 3 in, 3 out]
    }
  }
  n496 = while {
    shift-right: [w957] -> w93
    shift-left: w74 -> [w958]
    shift-right: [w959] -> w100
    shift-left: w101 -> [w960]
    tunnel: w96 -> [w956]
    tunnel: w95 -> [w955]
    tunnel: w40 -> [w954]
    tunnel: [w948] -> _
    tunnel: w82 -> [w947]
    tunnel: w72 -> [w946]
    tunnel: w7 -> [w945]
    stop <- "stop" stop-if-true
    n497 = event shown="[0] Timeout" {
      selector: _ -> [_ _ _ _ _ _ _ _ _ _ _ _ _ _ _]
      dyn-events: _ -> [_ _ _ _ _ _ _ _ _ _ _ _ _ _ _]
      timeout: 10 -> [_ _ _ _ _ _ _ _ _ _ _ _ _ _ _]
      tunnel: w960 -> [w971 w1017 w1027 w1041 w1112 w1116 w1120 w1160 w1176 w1193 w1236 w1253 w1269 w1279 w1290]
      tunnel: [w970 w1017 w1027 w1041 w1112 w1116 w1120 w1160 w1176 w1193 w1236 w1253 w1269 w1279 w1290] -> w959
      tunnel: w958 -> [w969 w1016 w1026 w1039 w1111 w1118 w1122 w1161 w1175 w1192 w1237 w1255 w1273 w1283 w1292]
      tunnel: [w968 w1016 w1026 w1038 w1113 w1118 w1121 _ w1175 w1192 w1237 w1254 w1272 w1282 w1291] -> w957
      tunnel: w956 -> [w967 _ _ _ _ _ _ _ _ _ _ _ _ _ _]
      tunnel: w955 -> [w966 _ _ _ _ _ _ _ _ _ _ _ _ _ _]
      tunnel: w954 -> [w965 _ _ _ _ _ _ _ _ _ _ _ _ _ _]
      tunnel: [w963 w1015 w1025 w1040 w1114 w1117 w1119 w1159 w1174 w1191 w1235 w1252 w1270 w1280 _] -> w948
      tunnel: w947 -> [w963 w1015 w1028 w1040 w1114 w1117 w1119 w1159 w1174 w1191 w1235 w1252 w1270 w1280 _]
      tunnel: w946 -> [_ _ _ _ _ _ _ _ _ _ _ w1256 w1271 w1284 w1289]
      tunnel: [_ _ _ _ _ _ _ w1161 _ _ _ _ _ _ _] -> _
      tunnel: w945 -> [w962 _ _ _ _ _ _ _ _ _ _ _ _ _ _]
      event Timeout {
        n498 = event-data() -> ()  [unwired: 1 in, 3 out]
        n499 = case shown="True" "Measuring" {
          tunnel: w971 -> [w973 w996]
          tunnel: [w973 w995] -> w970
          tunnel: w969 -> [w972 _]
          tunnel: [w972 w994] -> w968
          tunnel: w967 -> [_ w987]
          tunnel: w966 -> [_ w986]
          tunnel: w965 -> [_ w982]
          tunnel: w962 -> [_ w976]
          frame False {
          }
          frame True {
            w985 = ":FETCh? " ("data")
            w988 = u32 1000 ("byte count")
            # "Generate the data here."
            n500 = case shown="No Error" w982 {
              selector: w982 -> [w1008 w1009]
              tunnel: [w1008 w1009] -> w981
              tunnel: [w1007 _] -> w980
              frame No Error {
                n501 = Get Date/Time In Seconds() -> (seconds since 1Jan1904=w1007:timestamp)
              }
              frame Error {
              }
            }
            n502 = VISA Write(VISA resource name=w987, write buffer=w985, error in (no error)=w981) -> (VISA resource name out=w993:refnum<visa-resource-name>, error out=w991:errorcluster)  [unwired: 1 out]
            n503 = VISA Write(VISA resource name=w986, write buffer=w985, error in (no error)=w991) -> (VISA resource name out=w992:refnum<visa-resource-name>, error out=w990:errorcluster)  [unwired: 1 out]
            n504 = VISA Read(VISA resource name=w993, byte count=w988, error in (no error)=w990) -> (read buffer=w983:string, error out=w989:errorcluster)  [unwired: 2 out]
            n505 = VISA Read(VISA resource name=w992, byte count=w988, error in (no error)=w989) -> (read buffer=w984:string, error out=w978:errorcluster)  [unwired: 2 out]
            n506 = case shown="False" "DaQ" {
              tunnel: w978 -> [w998 w1004]
              tunnel: [w998 w1003] -> w977
              tunnel: w976 -> [_ w1002]
              tunnel: [0.0 ("Output") w1000] -> w974
              frame False {
              }
              frame True {
                n507 = local read "Number of Samples"() -> (w1006:i32)
                n508 = call-poly <vilib>:"DAQmx Read.vi"("task/channels in"=w1002, "number of samples per channel"=w1006, "error in"=w1004) -> ("data"=w1005:dbl[], "error out"=w1003:errorcluster)  [unwired: 10 in, 1 out]
                n509 = call-poly <vilib>:"Mean.vi"("X"=w1005) -> ("mean"=w1001:dbl)  [unwired: 1 out]
                "Actual mean" <- w1001
                n510 = call "N Point Running Average.vi"("n"="Moving average", "Input"=w1001) -> ("Output"=w1000:dbl)
              }
            }
            n511 = Bundle("seconds since 1Jan1904"=w980, "read buffer"=w983, "read buffer"=w984, "Output"=w974) -> (w979:T4)  [unwired: 1 in]
            n512 = Enqueue Element(queue=w996, element=w979, error in (no error)=w977) -> (queue out=w995:refnum<queue>, error out=w994:errorcluster)  [unwired: 1 in, 1 out]
          }
        }
      }
      event "Max Field (T)": Value Change {
        n513 = event-data() -> ()  [unwired: 1 in, 6 out]
        n514 = Divide(x="Max Field (T)", y="dB (T)") -> (x/y=w1012:dbl)
        n515 = for {
          N: w1012 -> [_]
          tunnel: "dB (T)" -> [w1022]
          tunnel: [w1019] -> w1011 mode=indexing
          tunnel: "Min Field (T)" -> [w1020]
          tunnel: [0.0] -> _ mode=indexing
          i -> [w1023]
          n516 = Multiply(x=w1023, y=w1022) -> (x*y=w1021:dbl)
          n517 = Add(x=w1021, y=w1020) -> (x+y=w1019:dbl)
        }
        "B array" <- w1011
      }
      event "Sweep Rate (T/min)": Value Change {
        n518 = event-data() -> ("NewVal"=w1029:dbl)  [unwired: 1 in, 5 out]
        n519 = local read "Magnet"() -> (w1024:bool)
        n520 = case shown="False" w1024 {
          tunnel: w1029 -> [_ w1036]
          tunnel: w1028 -> [w1030 w1032]
          tunnel: [w1030 w1031] -> w1025
          frame False {
          }
          frame True {
            n521 = Number To Fractional String(number=w1036, precision (6)=i16 3) -> (F-format string=w1034:string)  [unwired: 2 in]
            n522 = Concatenate Strings("T" ("format string"), w1034) -> (w1033:string)
            n523 = call "GPIB - BusCommand.vi"("Command"=w1033, "Address"=w1032) -> ("Address(thru)"=w1031:T6)  [unwired: 1 out]
          }
        }
      }
      event "Field To Zero": Value Change {
        n524 = event-data() -> ()  [unwired: 1 in, 6 out]
        n525 = Two Button Dialog(message="Do you want to switch off the field?", 1:"No" ("F button name (\"Cancel\")"), 2:"Yes" ("T button name (\"OK\")")) -> (T button?=w1045:bool)
        n526 = case shown="True" w1045 {
          tunnel: w1040 -> [_ w1050]
          tunnel: w1039 -> [w1046 w1048]
          tunnel: [w1046 w1047] -> w1038
          frame False {
          }
          frame True {
            n527 = local read "Magnet"() -> (w1049:bool)
            n528 = case shown="False" w1049 {
              tunnel: w1050 -> [_ w1102]
              tunnel: w1048 -> [w1053 w1099]
              tunnel: [w1052 w1099] -> w1047
              frame False {
                n529 = local read "Lock_in_Amplifier"() -> (w1051:refnum<visa-resource-name>)
                n530 = stacked-sequence {
                  seq-local: [w1056 _] -> [_ w1068]
                  seq-local: [w1054 _] -> [_ w1065]
                  tunnel: w1053 -> [w1058 _]
                  tunnel: [_ w1071] -> w1052
                  tunnel: w1051 -> [w1055 w1066]
                  frame #0 {
                    n531 = VISA Write(VISA resource name=w1055, write buffer="AUXV?1", error in (no error)=w1058) -> (VISA resource name out=w1062:refnum<visa-resource-name>, error out=w1057:errorcluster)  [unwired: 1 out]
                    n532 = VISA Read(VISA resource name=w1062, byte count=u32 1000, error in (no error)=w1057) -> (read buffer=w1059:string, error out=w1056:errorcluster)  [unwired: 2 out]
                    n533 = Fract/Exp String To Number(string=w1059) -> (number=w1054:dbl)  [unwired: 3 in, 1 out]
                  }
                  frame #1 {
                    w1074 = 0.001 ("Voltage Step (V)")
                    n534 = local read "Sweep Rate (T/min)"() -> (w1073:dbl)
                    n535 = local read "V/I (Ohm)"() -> (w1070:dbl)
                    n536 = local read "B/V (T/V)"() -> (w1064:dbl)
                    n537 = xnode "Sweep Delay"("SweepRate"=w1073, "Resolution"=w1074, "BpV"=w1064) -> ("Result"=w1072:dbl)  [unwired: 1 in, 1 out]
                    n538 = call "Universal_Ramping.vi"("milliseconds to wait"=w1072, "Initial Voltage (V)"=w1065, "error in (no error)"=w1068, "Voltage Step (V)"=w1074, "Final Voltage (V)"=0.0, "VISA resource name"=w1066) -> ("error out"=w1071:errorcluster, "Actual Voltage (V)"=w1063:dbl)  [unwired: 3 in, 1 out]
                    n539 = local write "Actual Voltage (V)"(w1063) -> ()
                    n540 = xnode "AUXtoB"("BpV"=w1064, "Rm"=w1070, "Aux"=w1063) -> ("Result"=w1069:dbl)  [unwired: 1 in, 1 out]
                    n541 = local write "Actual B Field (T)"(w1069) -> ()
                  }
                }
              }
              frame True {
                n542 = local read "Sweep Rate (T/min)"() -> (w1101:dbl)
                n543 = call "ips_switchHeaterOff.vi"("Instrument address"=w1102, "Rate"=w1101) -> ("B"=w1100:dbl)
                n544 = local write "Actual Field (T)"(w1100) -> ()
              }
            }
          }
        }
      }
      event "Go to Set": Value Change {
        n545 = event-data() -> ()  [unwired: 1 in, 6 out]
        n546 = local read "V/I (Ohm)"() -> (w1109:dbl)
        n547 = local read "B/V (T/V)"() -> (w1108:dbl)
        n548 = local read "Lock_in_Amplifier"() -> (w1105:refnum<visa-resource-name>)
        n549 = local read "Sweep Rate (T/min)"() -> (w1107:dbl)
        n550 = local read "Magnet"() -> (w1110:bool)
        n551 = call "Ramp_Field.vi"("Set Field (T) in"="Set Field (T)", "Sweep Rate (T/min)"=w1107, "V/I (Ohm)"=w1109, "error in (no error)"=w1111, "Magnet"=w1110, "B/V (T/V)"=w1108, "VISA Refnum in"=w1105) -> ("error out"=w1113:errorcluster, "Actual Voltage (V)"=w1103:dbl, "Set Field (T) out"=w1106:dbl)  [unwired: 2 in]
        n552 = local write "Actual B Field (T)"(w1106) -> ()
        n553 = local write "Actual Voltage (V)"(w1103) -> ()
      }
      event "Measure /Pause": Value Change {
        n554 = event-data() -> ("NewVal"=w1115:bool)  [unwired: 1 in, 5 out]
        n555 = local write "Measuring"(w1115) -> ()
      }
      event "Stop": Value Change {
        n556 = event-data() -> ()  [unwired: 1 in, 6 out]
        n557 = local read "Measuring"() -> (w1123:bool)
        n558 = case shown="True" w1123 {
          tunnel: w1122 -> [w1124 w1127]
          tunnel: [w1124 w1128] -> w1121
          frame False {
          }
          frame True {
            w1135 = FALSE ("Measuring")
            n559 = local read "SaveSweep"() -> (w1136:bool)
            n560 = local write "Measuring"(w1135) -> ()
            n561 = local write "Measure /Pause"(w1135) -> ()
            n562 = local read "Lock_in_Amplifier"() -> (w1129:refnum<visa-resource-name>)
            n563 = case shown="True" w1136 {
              frame False {
              }
              frame True {
                w1142 = 1 ("index (row)")
                w1143 = 0 ("index (row)")
                n564 = local read "Measurement File_average"() -> (w1155:path)
                n565 = local read "Averaged P(B)"() -> (w1144:dbl[][])
                n566 = local read "Averaged dt"() -> (w1146:dbl[][])
                n567 = local read "I(B) /Averaged/"() -> (w1154:cluster{"B array":dbl[], dbl[]}[])
                n568 = Index Array(array=w1146, index (row)=w1143) -> (element=w1145:dbl[])  [unwired: 1 in]
                n569 = Index Array(array=w1146, index (row)=w1142) -> (element=w1138:dbl[])  [unwired: 1 in]
                n570 = Index Array(array=w1154, index=1) -> (element=w1150:cluster{"B array":dbl[], dbl[]})
                n571 = Index Array(array=w1154, index=0) -> (element=w1151:cluster{"B array":dbl[], dbl[]})
                n572 = Unbundle(w1150) -> ("B array"=w1140:dbl[], w1139:dbl[])
                n573 = Unbundle(w1151) -> ("B array"=w1149:dbl[], w1148:dbl[])
                n574 = Index Array(array=w1144, index (row)=w1143) -> (element=w1141:dbl[])  [unwired: 1 in]
                n575 = Index Array(array=w1144, index (row)=w1142) -> (element=w1137:dbl[])  [unwired: 1 in]
                n576 = Build Array(w1149, w1148, w1145, w1141, w1140, w1139, w1138, w1137) -> (w1147:dbl[][])
                n577 = call-poly <vilib>:"Write Delimited Spreadsheet.vi"("file path (dialog if empty)"=w1155, "format (%.3f)"="%.5g", "2D data"=w1147, "append to file? (F)"=TRUE ("transpose? (F)"), "transpose? (F)"=TRUE ("append to file? (F)")) -> ()  [unwired: 9 in, 2 out]
              }
            }
            n578 = local read "V/I (Ohm)"() -> (w1133:dbl)
            n579 = local read "Sweep Rate (T/min)"() -> (w1132:dbl)
            n580 = local read "Set Field (T)"() -> (w1134:dbl)
            n581 = local read "B/V (T/V)"() -> (w1130:dbl)
            n582 = local read "Magnet"() -> (w1131:bool)
            n583 = call "Ramp_Field.vi"("Set Field (T) in"=w1134, "Sweep Rate (T/min)"=w1132, "V/I (Ohm)"=w1133, "error in (no error)"=w1127, "Magnet"=w1131, "B/V (T/V)"=w1130, "VISA Refnum in"=w1129) -> ("error out"=w1128:errorcluster, "Actual Voltage (V)"=w1125:dbl, "Set Field (T) out"=w1126:dbl)  [unwired: 2 in]
            n584 = local write "Actual B Field (T)"(w1126) -> ()
            n585 = local write "Actual Voltage (V)"(w1125) -> ()
          }
        }
      }
      event "Sweep": Value Change {
        n586 = event-data() -> ("NewVal"=w1162:bool)  [unwired: 1 in, 5 out]
        n587 = case shown="True" w1162 {
          frame False {
          }
          frame True {
            n588 = local read "Measurement File"() -> (w1163:path)
            n589 = Two Button Dialog(message="Do you want to create additional files for the sweeping measurements?" ("string"), 1:"No" ("F button name (\"Cancel\")"), 2:"Yes" ("T button name (\"OK\")")) -> (T button?=w1165:bool)
            n590 = case shown="True" w1165 {
              tunnel: w1163 -> [_ w1170]
              frame False {
                n591 = local write "SaveSweep"(FALSE ("SaveSweep")) -> ()
              }
              frame True {
                n592 = call "Create_sweep_files.vi"("Measurement File"=w1170) -> ("Path 3"=→"Measurement File_dn":path, "Path 2"=→"Measurement File_up":path, "Path"=→"Measurement File_average":path)  [unwired: 8 in]
                "SaveSweep" <- TRUE
              }
            }
          }
        }
      }
      event "Measure Noise": Value Change {
        n593 = event-data() -> ("NewVal"=w1177:bool)  [unwired: 1 in, 5 out]
        n594 = case shown="True" w1177 {
          frame False {
          }
          frame True {
            n595 = local read "Gain (V/A)"() -> (w1182:dbl)
            n596 = call "Noise_measurement.vi"("Gain (V/A)"=w1182, "Cycles"="Cycles", "Lower Cut-Off"="Cut-Off Frequency", "minimum value"="minimum value", "Filter On"="Filter On", "maximum value"="maximum value", "physical channels"="physical channels", "rate"="Rate", "samples per channel"="Samples per channel") -> ("Current (pA) Filtered"=→"Current (pA) Filtered":waveform(dbl), "PSD (pA/Hz^1/2) Peaks Removed"=→"PSD (pA/Hz^1/2) Peaks Removed":cluster{"f0":dbl, "df":dbl, "magnitude":dbl[]}, "Current (pA)"=→"Current (pA)":dbl[], "PSD (pA/Hz^1/2)"=→"PSD (pA/Hz^1/2)":cluster{"f0":dbl, "df":dbl, "magnitude":dbl[]})  [unwired: 3 in]
          }
        }
      }
      event "Calibrate": Value Change {
        n597 = event-data() -> ()  [unwired: 1 in, 6 out]
        n598 = case shown="True" "Calibrate" {
          frame False {
          }
          frame True {
            w1197 = dbl[] []
            n599 = while {
              shift-right: [w1230] -> w1195
              shift-left: dbl[][] [] -> [w1229]
              shift-right: [w1213] -> _
              shift-left: w1197 -> [w1225]
              shift-right: [w1222] -> _
              shift-left: w1197 -> [w1224]
              shift-right: [w1212] -> _
              shift-left: w1197 -> [w1223]
              shift-right: [w1204] -> _
              shift-left: 0.0 ("Set Field out") -> [w1203]
              stop <- w1226 stop-if-true
              n600 = call "Calibtarion.vi"("Dwell Time (ms)"="Dwell Time (ms)", "V array in (V)"=w1225, "I array in (A)"=w1223, "Collected array in"=w1229, "B array in (T)"=w1224, "Set Field (T)"=w1203, "dB"="dB") -> ("Best Linear Fit"=w1214:dbl[], "appended array"=→"appended array":dbl[][], "slope"=→"B/V (T/V)":dbl, "V array out (V)"=w1213:dbl[], "Boolean"=w1228:bool, "I array out (A)"=w1212:dbl[], "intercept 2"=→"I0 (A)":dbl, "Collected array out"=w1230:dbl[][], "intercept"=→"B0 (T)":dbl, "B array Out"=w1222:dbl[], "slope 2"=→"V/I (Ohm)":dbl, "Best Linear Fit 2"=w1219:dbl[], "Set Field out"=w1204:dbl)
              n601 = Bundle("I array out (A)"=w1212, "V array out (V)"=w1213) -> (w1221:T11)  [unwired: 1 in]
              n602 = Bundle("I array out (A)"=w1212, "Best Linear Fit"=w1214) -> (w1215:T12)  [unwired: 1 in]
              n603 = Bundle("V array out (V)"=w1213, "B array Out"=w1222) -> (w1217:T13)  [unwired: 1 in]
              n604 = Bundle("V array out (V)"=w1213, "Best Linear Fit 2"=w1219) -> (w1218:T14)  [unwired: 1 in]
              n605 = Or(x=w1228, y="stop 2") -> (x .or. y?=w1226:bool)
              n606 = Build Array(w1221, w1215) -> (→"V_I":T15)
              n607 = Build Array(w1217, w1218) -> (→"B_V":T16)
            }
            n608 = flat-sequence {
              tunnel: w1195 -> [w1201]
              frame #0 {
                n609 = Two Button Dialog(message="Do you want to save calibration file?") -> (T button?=w1200:bool)  [unwired: 2 in]
                n610 = case shown="True" w1200 {
                  tunnel: w1201 -> [_ w1202]
                  frame False {
                  }
                  frame True {
                    n611 = call-poly <vilib>:"Write Delimited Spreadsheet.vi"("2D data"=w1202) -> ()  [unwired: 13 in, 2 out]
                  }
                }
              }
            }
          }
        }
      }
      event "New Measurement File": Value Change {
        n612 = event-data() -> ()  [unwired: 1 in, 6 out]
        n613 = local read "Sweep"() -> (w1232:bool)
        n614 = Open/Create/Replace File(prompt="Please select measurement file\n", operation (0:open)=T5."replace or create with confirmation") -> (refnum out=w1238:refnum<file>)  [unwired: 4 in, 2 out]
        n615 = local write "refnum out"(w1238) -> ()
        n616 = Refnum to Path(1:w1238) -> (0:w1233:path)
        n617 = case shown="True" w1232 {
          tunnel: w1233 -> [_ w1241]
          frame False {
          }
          frame True {
            n618 = Two Button Dialog(message="Do you want to create additional files for the sweeping measurements?" ("string"), 1:"No" ("F button name (\"Cancel\")"), 2:"Yes" ("T button name (\"OK\")")) -> (T button?=w1243:bool)
            n619 = case shown="False" w1243 {
              tunnel: w1241 -> [_ w1251]
              frame False {
                n620 = local write "SaveSweep"(FALSE ("SaveSweep")) -> ()
              }
              frame True {
                n621 = call "Create_sweep_files.vi"("Measurement File"=w1251) -> ("Path 3"=w1248:path, "Path 2"=w1249:path, "Path"=w1250:path)  [unwired: 8 in]
                n622 = local write "Measurement File_dn"(w1248) -> ()
                n623 = local write "Measurement File_average"(w1250) -> ()
                n624 = local write "Measurement File_up"(w1249) -> ()
                n625 = local write "SaveSweep"(TRUE) -> ()
              }
            }
          }
        }
        n626 = local write "Measurement File"(w1233) -> ()
        n627 = local write "Offset?"(FALSE ("Offset?")) -> ()
        n628 = local write "First?"(TRUE ("First?")) -> ()
      }
      event "Heater On/Off": Value Change {
        n629 = event-data() -> ()  [unwired: 1 in, 6 out]
        n630 = case shown="False" "Heater On/Off" {
          tunnel: w1256 -> [w1261 w1267]
          tunnel: w1255 -> [w1259 w1268]
          tunnel: [w1258 w1266] -> w1254
          frame False {
            n631 = VISA Write(VISA resource name=w1261, write buffer="RANGE,1,0", error in (no error)=w1259) -> (error out=w1258:errorcluster)  [unwired: 2 out]
          }
          frame True {
            n632 = Number To Decimal String(number="Heater Range") -> (decimal integer string=w1264:string)  [unwired: 1 in]
            n633 = Concatenate Strings("RANGE,1," ("write buffer"), w1264) -> (w1262:string)
            n634 = VISA Write(VISA resource name=w1267, write buffer=w1262, error in (no error)=w1268) -> (error out=w1266:errorcluster)  [unwired: 2 out]
          }
        }
      }
      event "Set temperature (K)": Value Change {
        n635 = event-data() -> ()  [unwired: 1 in, 6 out]
        n636 = local read "Set temperature (K)"() -> (w1274:dbl)
        n637 = Number To Fractional String(number=w1274, precision (6)=i16 3) -> (F-format string=w1277:string)  [unwired: 2 in]
        n638 = Concatenate Strings("SETP 1," ("write buffer"), w1277) -> (w1275:string)
        n639 = VISA Write(VISA resource name=w1271, write buffer=w1275, error in (no error)=w1273) -> (error out=w1272:errorcluster)  [unwired: 2 out]
      }
      event "Temp Ramping Rate (K/min)": Value Change {
        n640 = event-data() -> ()  [unwired: 1 in, 6 out]
        n641 = local read "Temp Ramping Rate (K/min)"() -> (w1281:dbl)
        n642 = Number To Fractional String(number=w1281, precision (6)=i16 1) -> (F-format string=w1287:string)  [unwired: 2 in]
        n643 = Concatenate Strings("RAMP 1,1," ("string"), w1287) -> (w1286:string)
        n644 = VISA Write(VISA resource name=w1284, write buffer=w1286, error in (no error)=w1283) -> (error out=w1282:errorcluster)  [unwired: 2 out]
      }
      event "Heater Range": Value Change {
        n645 = event-data() -> ()  [unwired: 1 in, 6 out]
        n646 = local read "Heater On/Off"() -> (w1293:bool)
        n647 = case shown="True" w1293 {
          tunnel: w1292 -> [w1294 w1299]
          tunnel: [w1294 w1298] -> w1291
          tunnel: w1289 -> [_ w1297]
          frame False {
          }
          frame True {
            n648 = local read "Heater Range"() -> (w1295:enum16{"Off", "Low", "Medium", "High"})
            n649 = Number To Decimal String(number=w1295) -> (decimal integer string=w1301:string)  [unwired: 1 in]
            n650 = Concatenate Strings("RANGE,1," ("write buffer"), w1301) -> (w1300:string)
            n651 = VISA Write(VISA resource name=w1297, write buffer=w1300, error in (no error)=w1299) -> (error out=w1298:errorcluster)  [unwired: 2 out]
          }
        }
      }
    }
    n652 = Reciprocal(x="Sampling rate (Hz)") -> (1/x=w952:dbl)
    n653 = Multiply(x=w952, y=1000.0) -> (x*y=w950:dbl)
    n654 = Wait Until Next ms Multiple(millisecond multiple=w950) -> ()  [unwired: 1 out]
  }
  n655 = local read "Max Field (T)"() -> (w62:dbl)
  n656 = local read "Min Field (T)"() -> (w64:dbl)
  n657 = local read "dB (T)"() -> (w63:dbl)
  n658 = Divide(x=w62, y=w63) -> (x/y=w65:dbl)
  n659 = for {
    N: w65 -> [_]
    tunnel: w63 -> [w1306]
    tunnel: [w1303] -> w25 mode=indexing
    tunnel: w64 -> [w1304]
    tunnel: [0.0] -> _ mode=indexing
    i -> [w1307]
    n660 = Multiply(x=w1307, y=w1306) -> (x*y=w1305:dbl)
    n661 = Add(x=w1305, y=w1304) -> (x+y=w1303:dbl)
  }
  n662 = local write "No pol"(TRUE ("No pol")) -> ()
  n663 = Multiply(x=w25, y=0.0) -> (x*y=w22:dbl[])
  n664 = Array Size(array=w22) -> (size(s)=w21:i32)
  n665 = Decrement(x=w21) -> (x-1=w20:i32)
  n666 = local write "B array"(w25) -> ()
  n667 = Array Subset(array=w22, length=w20) -> (w19:dbl[])  [unwired: 1 in]
  n668 = Build Array(w22, w22) -> (w23:dbl[][])
  n669 = local write "Averaged I(B)"(w23) -> ()
  n670 = Build Array(w19, w19) -> (w18:dbl[][])
  n671 = local write "Averaged P(B)"(w18) -> ()
  n672 = local write "Averaged dt"(w18) -> ()
  n673 = local read "Lake Shore"() -> (w75:refnum<visa-resource-name>)
  n674 = local read "IV converter"() -> (w91:refnum<visa-resource-name>)
  n675 = local read "Magnetic Field"() -> (w90:refnum<visa-resource-name>)
  n676 = VISA Close(VISA resource name=w91, error in (no error)=w93) -> (error out=w94:errorcluster)
  n677 = VISA Close(VISA resource name=w90, error in (no error)=w94) -> (error out=w92:errorcluster)
  n678 = Release Queue(queue=w100, error in (no error)=w92) -> (error out=w88:errorcluster)  [unwired: 1 in, 2 out]
  n679 = Merge Errors(w88, w87) -> (w89:errorcluster)
  n680 = VISA Close(VISA resource name=w75, error in (no error)=w89) -> (error out=w86:errorcluster)
  n681 = local read "refnum out"() -> (w84:refnum<file>)
  n682 = Close File(refnum=w84, error in=w86) -> (error out=w85:errorcluster)  [unwired: 1 out]
  n683 = call <vilib>:"Simple Error Handler.vi"("error in (no error)"=w85) -> ()  [unwired: 4 in, 5 out]
  "i" <- w55
  "j" <- w55
